vi "信号光谱9 - MoO3.vi"() -> ()   [LabVIEW 2018]
uses:
  <vilib>/Utility/NIReport.llb/Report Type.ctl
  <vilib>/Utility/file.llb/Write Delimited Spreadsheet (DBL).vi
  <vilib>/Instr/_visa.llb/VISA Configure Serial Port (Instr).vi
  <vilib>/addons/_office/excel.llb/Excel Get Data ([str]).vi
  <vilib>/Utility/NIReport.llb/NI_report.lvclass
  <vilib>/Analysis/NI_AALBase.lvlib
  <vilib>/ptbypt/NI_PtbyPt.lvlib
  <vilib>/Utility/NIReport.llb/NI_ReportGenerationCore.lvlib
  <vilib>/addons/_office/NI_ReportGenerationToolkit.lvlib
  <vilib>/Utility/NIReport.llb/Excel/NI_Excel.lvclass
panel:
  in  "判断角度上限":dbl=4.0 format="%#_13g"
  in  "判断角度下限":dbl=1.0 format="%#_13g"
  out "原始峰值":dbl
  out "拟合峰值":dbl
  in  "角度倍乘系数":dbl=1.5
  out "结果展示":dbl[][](array[numeric])=[[37.33100777239877, 2672.955043835526, 29.54153292599307, 222755.0, 50.0], [37.36593979472361, 2672.656498058864, 30.113284142729572, 222833.0, 50.0], [38.96986225690859, 2673.3337152325566, 33.38805102415213, 222910.0, 75.0], [37.39946104045098, 2676.4005085744548, 31.215565446104666, 222948.0, 47.0], [35.862209164247574, 2671.7826876859012, 30.355582265151796, 223028.0, 47.0]]
  out "Δw2>C":bool=TRUE
  out "Δw1>C":bool=TRUE
  out "θi":dbl
  in  "w0":dbl format="%#_13g"
  in  "C=w-w0":dbl=1800.0 format="%#_13g"
  in  "上升下降沿/s":dbl format="%.2p"
  in  "延时/s":dbl format="%.2p"
  in  "占空比/%":dbl=3.0 format="%.2p"
  in  "高电平/V":dbl=4.0 format="%.2p"
  in  "频率/Hz":dbl=6000.0 format="%.3p"
  in  "低电平/V":dbl min=0.0 max=5.0 format="%.2p"
  in  "Enable":bool
  in  "上升下降沿":i32(ring)=1 items=["上升沿", "下降沿"]
  in  "输出信号波形":u16(ring) items=["Pulse"]
  out "Output":bool
  in  "VISA 信号发生器":refnum<visa-resource-name>="USB0::0x1AB1::0x0641::DG4E192200870::INSTR"
  out "Output 2":bool
  in  "Enable 2":bool
  in  "上升下降沿/s 2":dbl format="%.2p"
  in  "延时/s 2":dbl format="%.2p"
  in  "占空比/% 2":dbl=3.0 format="%.2p"
  in  "高电平/V 2":dbl=0.002 format="%.2p"
  in  "频率/Hz 2":dbl=6000.0 format="%.3p"
  in  "低电平/V 2":dbl min=0.0 max=5.0 format="%.2p"
  in  "上升下降沿 2":i32(ring)=1 items=["上升沿", "下降沿"]
  in  "输出信号波形 2":u16(ring) items=["Pulse"]
  in  "终止测量":bool
  in  "测量次数":i32=1
  out "best fit":cluster{"Y":dbl[], "Y":dbl[]}[](graph)
  in  "拟合终点":i32=850
  in  "拟合起点":i32=200
  out "angle":dbl
  out "图片地址":string
  in  "开光时间/ms":u32=50
  out "最终存储路径 2":path
  out "照明光error out":errorcluster
  in  "照明光":bool
  in  "stop bits (10: 1 bit)":u16(ring)=10 items=["1.0"=10, "1.5"=15, "2.0"=20]
  in  "parity (0:none)":enum16{"None", "Odd", "Even", "Mark", "Space"}(ring)
  in  "data bits (8)":u16=8 min=5 max=8 step=1
  in  "baud rate":u32=9600 caption="baud rate (115200)" min=9600 max=115200
  in  "照明光VISA":refnum<visa-resource-name>="COM6"
  out "正在测量":bool
  in  "滤波阈值":dbl=300.0 format="%#_13g"
  out "范围内？":bool[](array[boolean])
  out "w":dbl
  out "xc":dbl
  out "拟合参数":dbl[](array[numeric])
  out "最终存储路径":path
  in  "停止程序":bool
  out "configure error out":errorcluster
  in  "设置参数":bool
  out "output control error  4":errorcluster
  in  "低电平持续输出":bool
  out "output control error  5":errorcluster
  out "output control error":errorcluster
  in  "开始测量":bool
  in  "channel输出口":i32(ring) items=["Channel 1", "Channel 2"]
  out "output control error":errorcluster
  out "Spectrum":cluster{"Y":dbl[], "Y":dbl[]}[](graph)
  out "波长范围":dbl[](array[numeric])
  in  "?":enum32{"IHR 550", "CCD"}(tab)
  in  "Move To\nTarget Positions":bool
  out "Current UniqueID":string="Mono4"
  in  "Mono ID":string(combo)="Mono1"
  in  "Connect":bool
  out "Initialized JY":bool=TRUE
  in  "Force\nInitialization":bool
  in  "Target Grating":string(combo)="2"
  out "Current Description":string="1" caption="Description"
  out "Grating Index":i32=1
  out "Current Grating":dbl=1200.0
  out "Units":string="nm"
  out "Current WL":dbl=897.9988
  out "Exit Mirror\nPosition":i32(ring)=2 items=["EntranceMirror", "ExitMirror", "Front", "Side"]
  out "Entrance Mirror\nPosition":i32(ring)=2 items=["EntranceMirror", "ExitMirror", "Front", "Side"]
  out "Units 2":string="mm"
  out "Front Entrance":dbl
  in  "Target WL":dbl=516.0
  in  "Exit Mirror":u16(ring)=3 caption="Target Position Exit Mirror" items=["Front"=2, "Side"=3]
  in  "Entrance Mirror":u16(ring)=2 caption="Target Position\nEntrance Mirror" items=["Front"=2, "Side"=3]
  in  "Target\nFront Entrance":dbl=2.0
  in  "Commande tab":T1(tab)
  in  "Area Number to Display":i32
  in  "Reformat":bool
  in  "GAIN":u16(ring)=2 caption="Device Name" items=["High Light", "Best Dynamic Range", "High Sensitivity"]
  in  "ADC":u16(ring) caption="Device Name" items=["20 kHz       ", " 1 MHz       ", " 1 MHz Ultra "]
  in  "Number of Areas :":u16=1 min=1 step=1
  in  "Integration time (ms) :":i16=20000
  out "Uniques ID":u16(ring) items=["CCD1", "CCD2"]
  in  "Device Name":u16(ring) items=["Synapse CCD (Lateral)", "Synapse_IGA (Axial)"]
  in  "Signal type :":enum16{"TTL Rising Edge", "TTL Falling Edge"}(ring)=enum."TTL Falling Edge"
  in  "Trigger Type :":u16(ring) items=["On Start"=1, "Per Acquisition"=2]
  in  "trigSigTypeString":string
  in  "trigEventString":string
  in  "Enable InputTriggers :":bool
  in  "Number of Cleans":i32=1
  in  "MultiAcqShutterMode":i32(ring)=3 items=["Open For All Spectra"=1, "Open for Each Spectrum"=3]
  in  "Accumulations:":u16=10 min=1 step=1
  in  "Multi Accumulation mode:":bool
  out "Y Pixels:":i32=256
  out "DataSize":i32=1024
  out "X Pixels:":i32=1024
  out "Firmware\nVersion":string="V1.20 CCD_4000"
  out "initialized ?":bool=TRUE
  in  "Continuous":bool
  in  "CCD Busy":bool
  out "indicator":string="Ready !"
  in  "initialize":bool
  in  "ShutterOpen":bool=TRUE caption="Shutter enable"
  in  "Acquire":bool
  in  "Temperature":bool
  in  "Setup":bool
  out "Acq Time(ms)":u32=3401
  in  "Save Backlight":bool
  in  "cut backlight":bool
  out "backlight":bool=TRUE
  in  "是否拟合":bool
  in  "是否保存":bool
  in  "Close":bool=TRUE
  out "JYCCDLib.IJYCCDReqd":refnum<k7>
  out "areas :":i32[][](array[numeric])=[[1], [1], [1], [1024], [256], [1], [256]]
  in  "Constante de condition\n(Voir l'aide contextuelle)":bool
  out "temp graph":dbl(graph)=-134.538067
  out "ADC Number":i32[](array[numeric])=[0, 1, 2, 3, 4]
  out "Gain Number":i32[](array[numeric])=[10, 11, 12, 13, 8, 2]
  out "trigAddress":i32
  out "Data":i32[][](graph)
  out "error out":errorcluster
  out "Gratings":dbl[](array[numeric])=[1200.0, 300.0]
  out "Backlight":i32[][](graph)
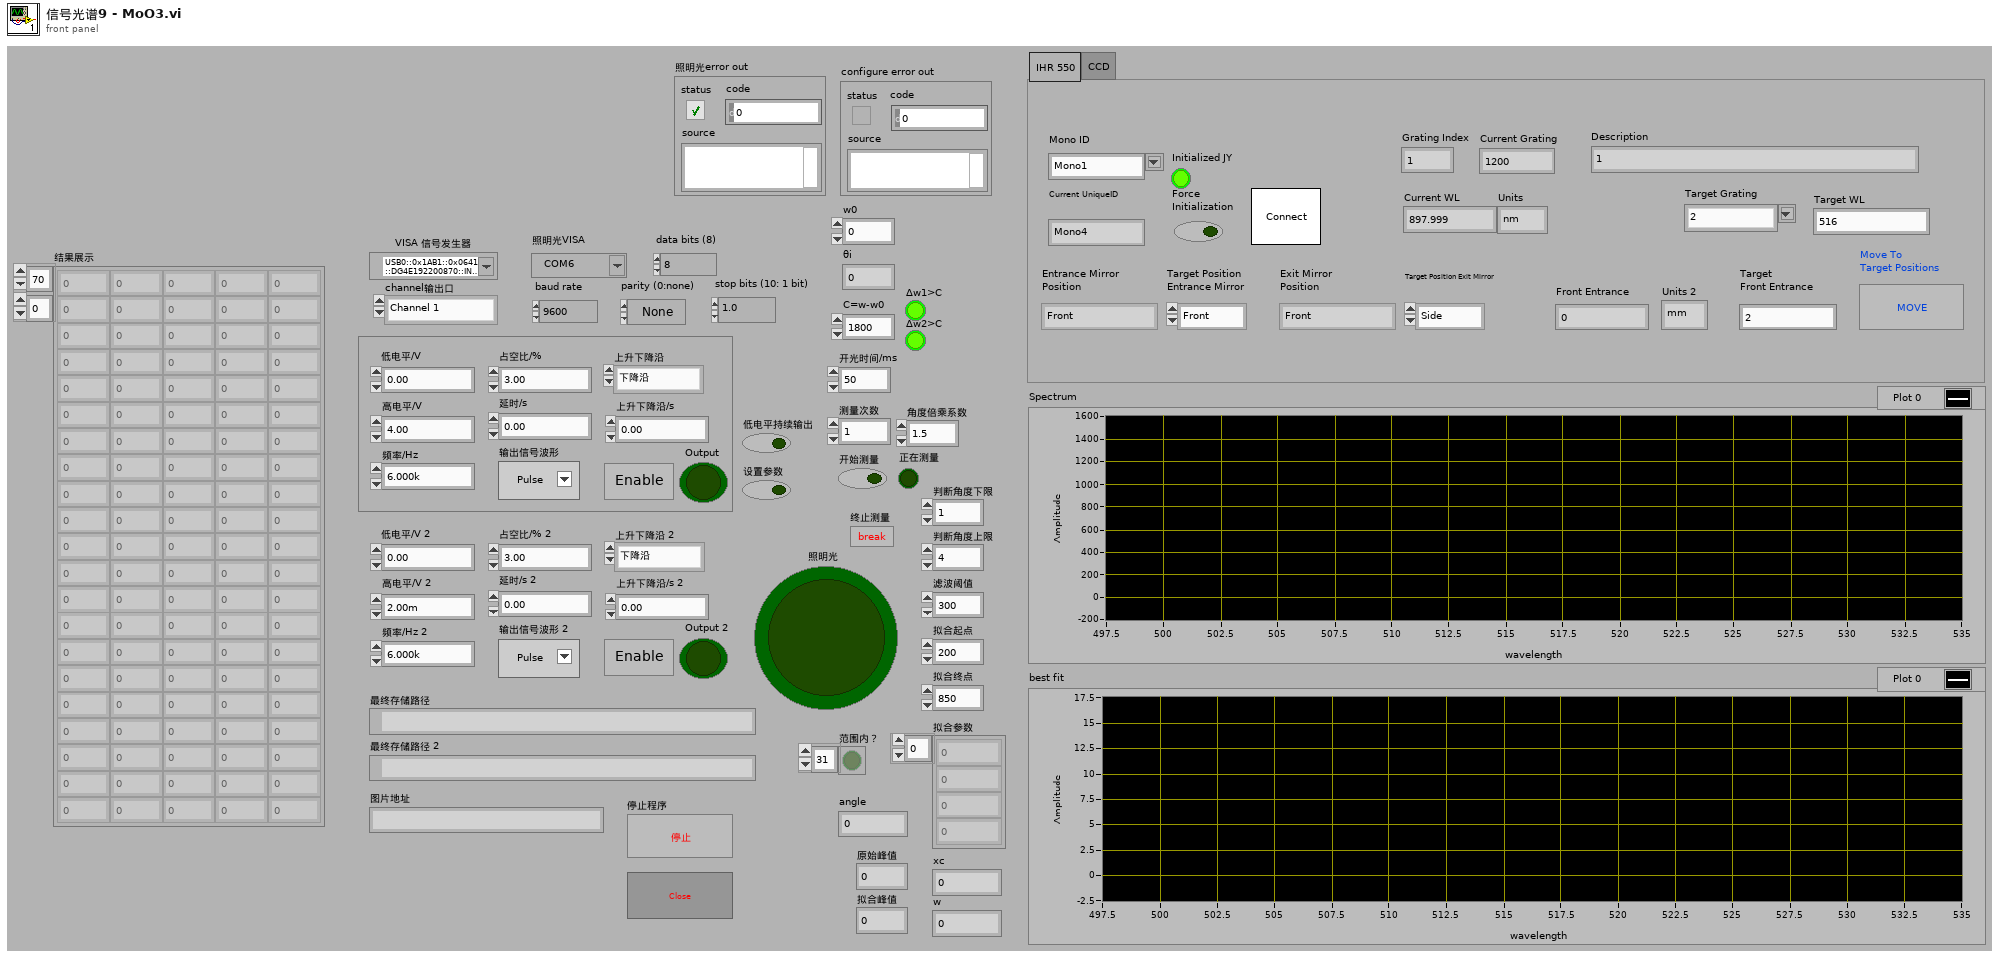
[diagram p1: front panel]
types:
  T1 = enum32{"Settings", "Trigger In", "Multi-Accu.", "Infos"}
  T2 = enum8{"Enabled", "Disabled", "Disabled and Grayed Out"}
  T3 = enum16{"maximized", "minimized", "normal", "no change"}
  T4 = typedef "NI_ReportGenerationCore.lvlib/Report Type.ctl" = enum16{"HTML", "Word", "Excel"}
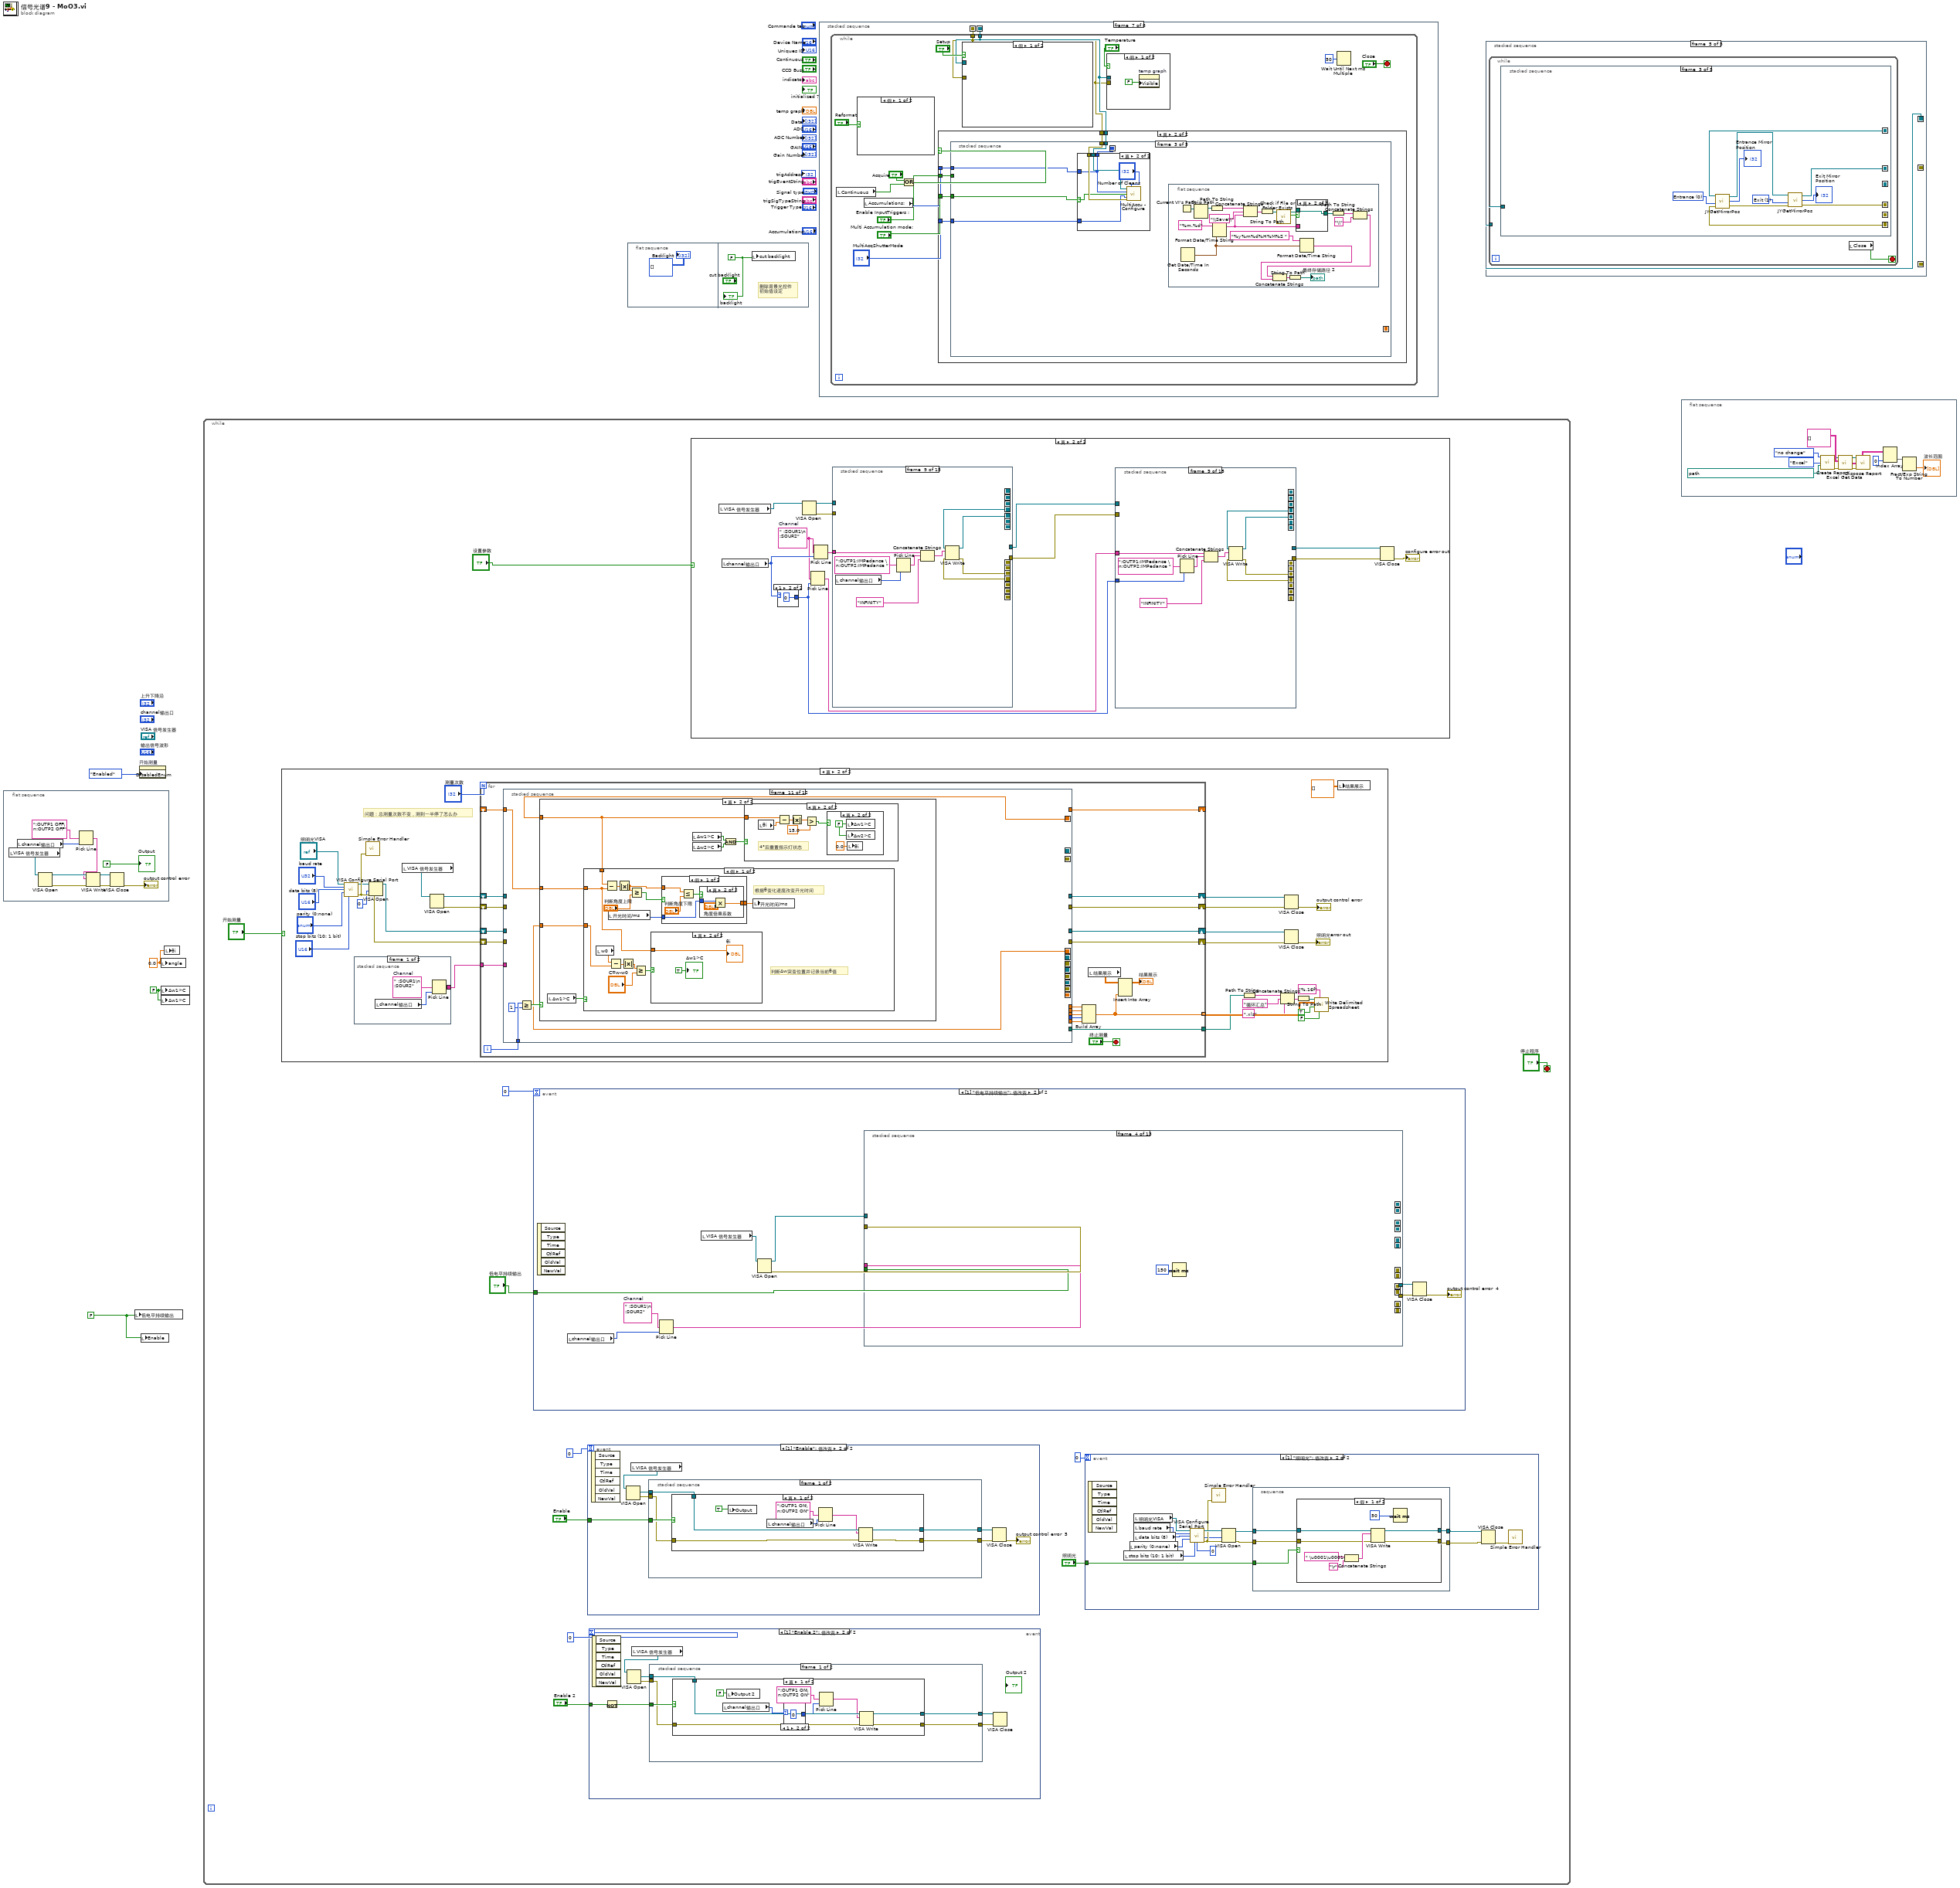
[diagram p0: block diagram]
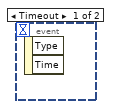
[diagram p2: hidden frame]
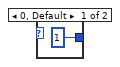
[diagram p3: hidden frame]
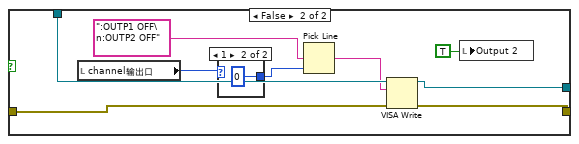
[diagram p4: hidden frame]
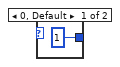
[diagram p5: hidden frame]
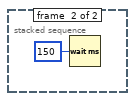
[diagram p6: hidden frame]
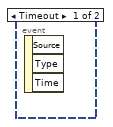
[diagram p7: hidden frame]
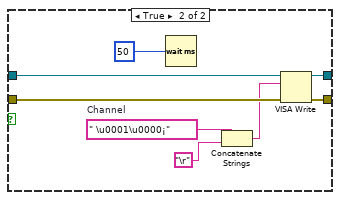
[diagram p8: hidden frame]
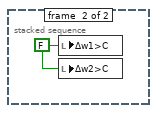
[diagram p10: hidden frame]
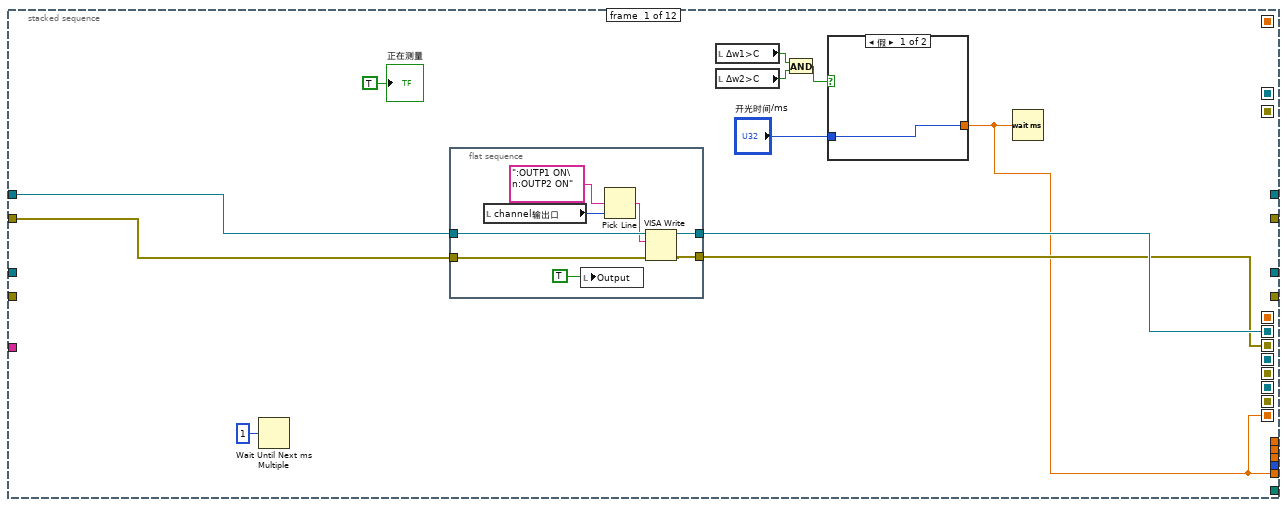
[diagram p11: hidden frame]
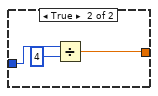
[diagram p12: hidden frame]
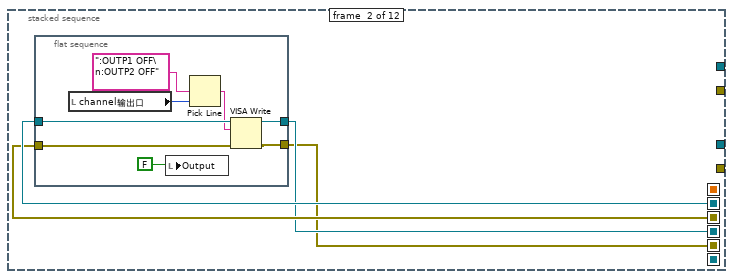
[diagram p13: hidden frame]
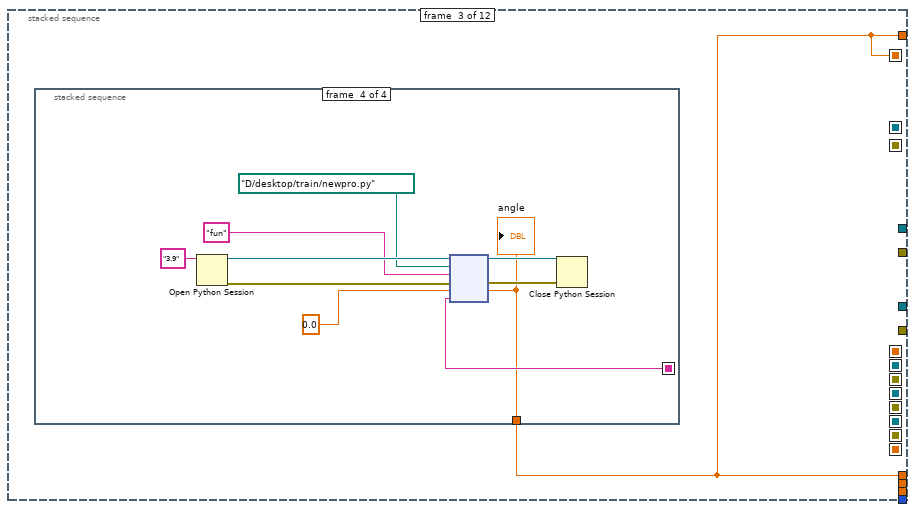
[diagram p14: hidden frame]
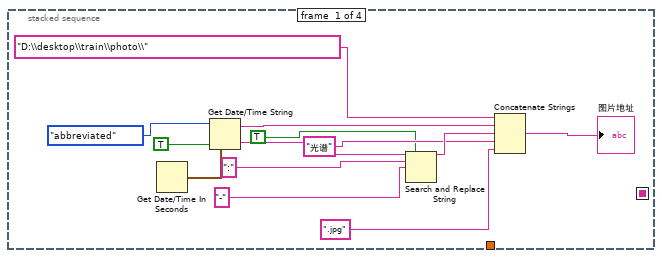
[diagram p15: hidden frame]
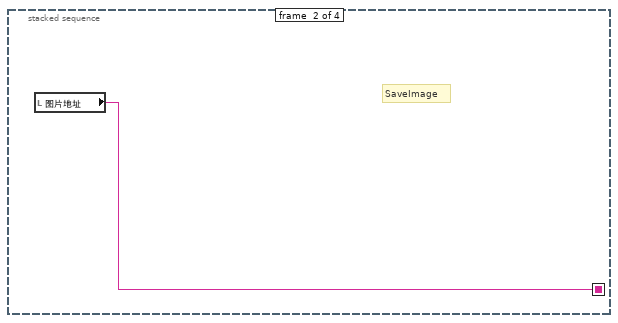
[diagram p16: hidden frame]
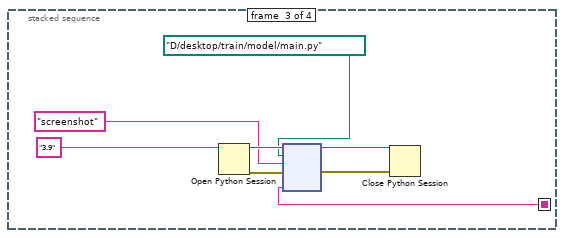
[diagram p17: hidden frame]
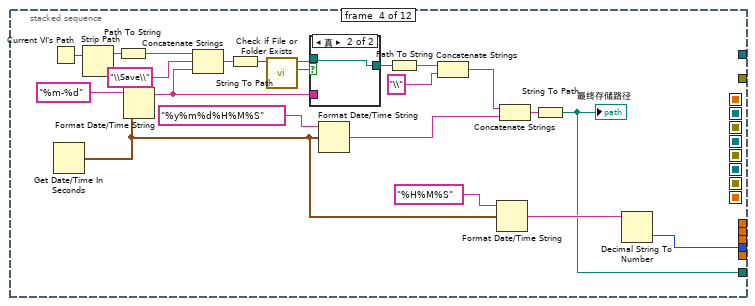
[diagram p18: hidden frame]
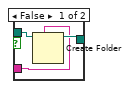
[diagram p19: hidden frame]
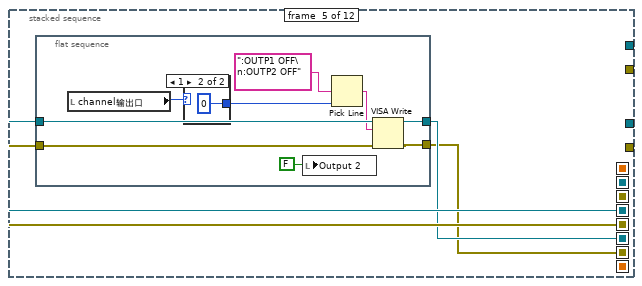
[diagram p20: hidden frame]
diagram:
  w1 = FALSE ("Δw1>C")
  w2 = 0.0 ("angle")
  w3 = FALSE
  n1 = flat-sequence {
    frame #0 {
      n2 = local read "VISA 信号发生器"() -> (w8:refnum<visa-resource-name>)
      n3 = local read "channel输出口"() -> (w6:i32)
      n4 = VISA Open(VISA resource name=w8) -> (VISA resource name=w14:refnum<visa-resource-name>, error out=w13:errorcluster)  [unwired: 4 in]
      n5 = Pick Line(multi-line string=":OUTP1 OFF\n:OUTP2 OFF" ("write buffer"), line index=w6) -> (output string=w5:string)  [unwired: 1 in]
      n6 = VISA Write(VISA resource name=w14, write buffer=w5, error in (no error)=w13) -> (VISA resource name out=w11:refnum<visa-resource-name>, error out=w10:errorcluster)  [unwired: 1 out]
      n7 = VISA Close(VISA resource name=w11, error in (no error)=w10) -> (error out=→"output control error":errorcluster)
      "Output" <- FALSE ("布尔")
    }
  }
  n8 = local write "低电平持续输出"(w3) -> ()
  n9 = property on="开始测量" class="Bool"("DisabledEnum"=T2."Enabled" ("禁用")) -> ()  [unwired: 2 in, 2 out]
  n10 = local write "Enable"(w3) -> ()
  n11 = local write "angle"(w2) -> ()
  n12 = local write "Δw1>C"(w1) -> ()
  n13 = local write "Δw1>C"(w1) -> ()
  n14 = local write "θi"(w2) -> ()
  n15 = while {
    stop <- "停止程序" stop-if-true
    n16 = case shown="真" "开始测量" {
      frame False {
      }
      frame True {
        # "问题：总测量次数不变，测到一半停了怎么办"
        n17 = call-poly "VISA Configure Serial Port"("VISA resource name"="照明光VISA", "baud rate (9600)"="baud rate", "data bits (8)"="data bits (8)", "parity (0:none)"="parity (0:none)", "stop bits (10: 1 bit)"="stop bits (10: 1 bit)") -> ("VISA resource name out"=w118:refnum<visa-resource-name>, "error out"=w119:errorcluster)  [unwired: 9 in]
        n18 = stacked-sequence {
          tunnel: [w128 _] -> w122
          frame #0 {
            w129 = " :SOUR1\n :SOUR2"  # Channel
            n19 = local read "channel输出口"() -> (w130:i32)
            n20 = Pick Line(multi-line string=w129, line index=w130) -> (output string=w128:string)  [unwired: 1 in]
          }
          frame #1 {
            w131 = FALSE ("Δw1>C")
            n21 = local write "Δw1>C"(w131) -> ()
            n22 = local write "Δw2>C"(w131) -> ()
          }
        }
        n23 = call <vilib>:"Simple Error Handler.vi"("error in (no error)"=w119) -> ()  [unwired: 4 in, 5 out]
        n24 = VISA Open(access mode=0, error in (no error)=w119, VISA resource name=w118) -> (VISA resource name=w111:refnum<visa-resource-name>, error out=w110:errorcluster)  [unwired: 2 in]
        n25 = local read "VISA 信号发生器"() -> (w127:refnum<visa-resource-name>)
        n26 = VISA Open(VISA resource name=w127) -> (VISA resource name=w126:refnum<visa-resource-name>, error out=w125:errorcluster)  [unwired: 4 in]
        n27 = for {
          N: "测量次数" -> [_]
          tunnel: w122 -> [w151]
          shift-right: [w147] -> w121
          shift-left: w126 -> [w153]
          shift-right: [w146] -> w120
          shift-left: w125 -> [w152]
          shift-right: [w145] -> w124
          shift-left: w111 -> [w150]
          shift-right: [w144] -> w123
          shift-left: w110 -> [w149]
          tunnel: [w134] -> w100 mode=indexing
          shift-right: [w139] -> _
          shift-left: _ -> [w138]
          tunnel: [w135] -> w97
          i -> [w137]
          stop <- "终止测量" stop-if-true
          n28 = stacked-sequence {
            seq-local: [w160 _ _ _ _ _ _ _ _ _ _ _] -> [_ w180 _ _ _ _ _ _ _ _ _ _]
            seq-local: [w159 _ _ _ _ _ _ _ _ _ _ _] -> [_ w179 _ _ _ _ _ _ _ _ _ _]
            seq-local: [_ _ _ _ _ w265 _ _ _ _ _ _] -> [_ _ _ _ _ _ _ _ w383 _ _ _]
            seq-local: [_ _ _ _ _ w264 _ _ _ _ _ _] -> [_ _ _ _ _ _ _ _ w386 _ _ _]
            seq-local: [_ w178 _ _ _ _ _ _ _ _ _ _] -> [_ _ _ _ w251 _ _ _ _ _ _ _]
            seq-local: [_ w177 _ _ _ _ _ _ _ _ _ _] -> [_ _ _ _ w250 _ _ _ _ _ _ _]
            seq-local: [_ _ _ _ w249 _ _ _ _ _ _ _] -> [_ _ _ _ _ _ _ w369 _ _ _ _]
            seq-local: [_ _ _ _ w248 _ _ _ _ _ _ _] -> [_ _ _ _ _ _ _ w368 _ _ _ _]
            seq-local: [_ _ w189 _ _ _ _ _ _ _ _ _] -> [_ _ _ _ _ _ _ _ _ _ w395 _]
            seq-local: [_ _ _ _ _ _ w280 _ _ _ _ _] -> [_ _ _ _ _ _ _ _ _ _ w390 _]
            seq-local: [w154 _ _ _ _ _ _ _ _ _ _ _] -> [_ _ _ _ _ _ w278 _ _ _ _ _]
            tunnel: w153 -> [w162 _ _ _ _ _ _ _ _ _ _ _]
            tunnel: w152 -> [w161 _ _ _ _ _ _ _ _ _ _ _]
            tunnel: [_ _ _ _ _ _ _ w367 _ _ _ _] -> w147
            tunnel: [_ _ _ _ _ _ _ w366 _ _ _ _] -> w146
            tunnel: w151 -> [_ _ _ _ _ _ _ _ _ _ _ _]
            tunnel: w150 -> [_ _ _ _ _ w268 _ _ _ _ _ _]
            tunnel: w149 -> [_ _ _ _ _ w267 _ _ _ _ _ _]
            tunnel: [_ _ _ _ _ _ _ _ w385 _ _ _] -> w145
            tunnel: [_ _ _ _ _ _ _ _ w384 _ _ _] -> w144
            tunnel: [_ _ w189 _ _ _ _ _ _ _ _ _] -> w143
            tunnel: [_ _ _ _ _ _ w275 _ _ _ _ _] -> w142
            tunnel: [_ _ _ _ _ _ w274 _ _ _ _ _] -> w141
            tunnel: [_ _ _ w223 _ _ _ _ _ _ _ _] -> w140
            tunnel: [w154 _ _ _ _ _ _ _ _ _ _ _] -> w136
            tunnel: [_ _ w189 _ _ _ _ _ _ _ _ _] -> w139
            tunnel: w138 -> [_ _ _ _ _ _ _ _ _ _ w394 _]
            tunnel: w137 -> [_ _ _ _ _ _ _ _ _ _ w392 _]
            tunnel: [_ _ _ w222 _ _ _ _ _ _ _ _] -> w135
            frame #0 {
              n29 = Wait Until Next ms Multiple(millisecond multiple=u32 1 ("毫秒倍数")) -> ()  [unwired: 1 out]
              n30 = flat-sequence {
                tunnel: w162 -> [w176]
                tunnel: w161 -> [w175]
                tunnel: [w170] -> w160
                tunnel: [w169] -> w159
                frame #0 {
                  n31 = local read "channel输出口"() -> (w172:i32)
                  n32 = local write "Output"(TRUE ("布尔")) -> ()
                  n33 = Pick Line(multi-line string=":OUTP1 ON\n:OUTP2 ON" ("write buffer"), line index=w172) -> (output string=w171:string)  [unwired: 1 in]
                  n34 = VISA Write(VISA resource name=w176, write buffer=w171, error in (no error)=w175) -> (VISA resource name out=w170:refnum<visa-resource-name>, error out=w169:errorcluster)  [unwired: 1 out]
                }
              }
              n35 = local read "Δw1>C"() -> (w156:bool)
              n36 = local read "Δw2>C"() -> (w157:bool)
              n37 = And(x=w156, y=w157) -> (x .and. y?=w155:bool)
              n38 = case shown="假" w155 {
                tunnel: [w165 w166] -> w154
                tunnel: "开光时间/ms" -> [w165 w168]
                frame False {
                }
                frame True {
                  n39 = Divide(x=w168, y=u32 4) -> (x/y=w166:dbl)
                }
              }
              n40 = Wait (ms)(milliseconds to wait=w154) -> ()  [unwired: 1 out]
              "正在测量" <- TRUE
            }
            frame #1 {
              n41 = flat-sequence {
                tunnel: w180 -> [w188]
                tunnel: w179 -> [w187]
                tunnel: [w182] -> w178
                tunnel: [w181] -> w177
                frame #0 {
                  n42 = local read "channel输出口"() -> (w184:i32)
                  n43 = local write "Output"(FALSE ("布尔")) -> ()
                  n44 = Pick Line(multi-line string=":OUTP1 OFF\n:OUTP2 OFF" ("write buffer"), line index=w184) -> (output string=w183:string)  [unwired: 1 in]
                  n45 = VISA Write(VISA resource name=w188, write buffer=w183, error in (no error)=w187) -> (VISA resource name out=w182:refnum<visa-resource-name>, error out=w181:errorcluster)  [unwired: 1 out]
                }
              }
            }
            frame #2 {
              n46 = stacked-sequence {
                seq-local: [_ w203 _ _] -> [_ _ w204 w213]
                tunnel: [_ _ _ w212] -> w189
                frame #0 {
                  n47 = Get Date/Time In Seconds() -> (seconds since 1Jan1904=w199:timestamp)
                  n48 = Get Date/Time String(date format (0)=enum16{"short", "long", "abbreviated"}."abbreviated" ("日期格式(0)"), seconds (now)=w199, want seconds? (F)=TRUE ("需要秒？(F)")) -> (date string=w202:string, time string=w200:string)
                  n49 = Search and Replace String(replace all?=TRUE ("替换全部？(F)"), input string=w200, search string=":" ("搜索字符串"), replace string="-" ("替换字符串(\"\")")) -> (result string=w201:string)  [unwired: 4 in, 3 out]
                  n50 = Concatenate Strings("D:\\desktop\\train\\photo\\", w202, w201, "光谱" ("字符串"), ".jpg" ("字符串")) -> (→"图片地址":string)
                }
                frame #1 {
                  # "SaveImage"
                  n51 = local read "图片地址"() -> (w203:string)
                }
                frame #2 {
                  n52 = Open Python Session(python version="3.9" ("Python version")) -> (session out=w211:refnum<k35>, error out=w209:errorcluster)  [unwired: 2 in]
                  n53 = node(w211, path "D:/desktop/train/model/main.py" ("module path"), "screenshot" ("function name"), w209, w204) -> (w210:refnum<k35>, w208:errorcluster)  [unwired: 3 in, 2 out]
                  n54 = Close Python Session(session in=w210, error in=w208) -> ()  [unwired: 1 out]
                }
                frame #3 {
                  n55 = Open Python Session(python version="3.9" ("Python version")) -> (session out=w220:refnum<k35>, error out=w218:errorcluster)  [unwired: 2 in]
                  n56 = node(w220, path "D:/desktop/train/newpro.py" ("module path"), "fun" ("function name"), w218, 0.0, w213) -> (w219:refnum<k35>, w217:errorcluster, w212:dbl)  [unwired: 1 in, 2 out]
                  "angle" <- w212
                  n57 = Close Python Session(session in=w219, error in=w217) -> ()  [unwired: 1 out]
                }
              }
            }
            frame #3 {
              n58 = Current VI's Path() -> (path=w232:path)
              n59 = Get Date/Time In Seconds() -> (seconds since 1Jan1904=w225:timestamp)
              n60 = Strip Path(path=w232) -> (stripped path=w233:path)  [unwired: 1 out]
              n61 = Path To String(path=w233) -> (string=w234:string)
              n62 = Format Date/Time String(time format string (%c)="%m-%d" ("时间格式字符串(%c)"), seconds (now)=w225) -> (date/time string=w240:string)  [unwired: 1 in]
              n63 = Concatenate Strings(w234, "\\Save\\" ("字符串"), w240) -> (w235:string)
              n64 = String To Path(string=w235) -> (path=w236:path)
              n65 = call <vilib>:"Check if File or Folder Exists.vi"("path"=w236) -> ("file or folder exists?"=w237:bool, "dup path"=w239:path)  [unwired: 8 in, 1 out]
              n66 = case shown="真" w237 {
                tunnel: [w246 w247] -> w238
                tunnel: w239 -> [w245 w247]
                tunnel: w240 -> [w244 _]
                frame False {
                  n67 = Create Folder(prompt (Create Folder)=w244, path (use dialog)=w245) -> (created path=w246:path)  [unwired: 1 in, 2 out]
                }
                frame True {
                }
              }
              n68 = Format Date/Time String(time format string (%c)="%y%m%d%H%M%S" ("时间格式字符串(%c)"), seconds (now)=w225) -> (date/time string=w243:string)  [unwired: 1 in]
              n69 = Path To String(path=w238) -> (string=w241:string)
              n70 = Concatenate Strings(w241, "\\" ("字符串")) -> (w242:string)
              n71 = Format Date/Time String(time format string (%c)="%H%M%S" ("时间格式字符串(%c)"), seconds (now)=w225) -> (date/time string=w224:string)  [unwired: 1 in]
              n72 = Concatenate Strings(w242, w243) -> (w231:string)
              n73 = String To Path(string=w231) -> (path=w222:path)
              "最终存储路径" <- w222
              n74 = Decimal String To Number(string=w224) -> (number=w223:i32)  [unwired: 2 in, 1 out]
            }
            frame #4 {
              n75 = flat-sequence {
                tunnel: w251 -> [w260]
                tunnel: w250 -> [w259]
                tunnel: [w255] -> w249
                tunnel: [w254] -> w248
                frame #0 {
                  n76 = local read "channel输出口"() -> (w253:i32)
                  n77 = case shown="1" w253 {
                    tunnel: [1 0] -> w252
                    frame 0, Default {
                    }
                    frame 1 {
                    }
                  }
                  n78 = local write "Output 2"(FALSE ("布尔")) -> ()
                  n79 = Pick Line(multi-line string=":OUTP1 OFF\n:OUTP2 OFF" ("write buffer"), line index=w252) -> (output string=w256:string)  [unwired: 1 in]
                  n80 = VISA Write(VISA resource name=w260, write buffer=w256, error in (no error)=w259) -> (VISA resource name out=w255:refnum<visa-resource-name>, error out=w254:errorcluster)  [unwired: 1 out]
                }
              }
            }
            frame #5 {
              w263 = " \u0001\u0001¢"  # Channel
              n81 = Wait (ms)(milliseconds to wait=1200) -> ()  [unwired: 1 out]
              n82 = Concatenate Strings(w263, "\r") -> (w269:string)
              n83 = local write "照明光"(FALSE ("照明光")) -> ()
              n84 = VISA Write(VISA resource name=w268, write buffer=w269, error in (no error)=w267) -> (VISA resource name out=w265:refnum<visa-resource-name>, error out=w264:errorcluster)  [unwired: 1 out]
            }
            frame #6 {
              n85 = local read "Area Number to Display"() -> (w319:i32)
              n86 = local read "JYCCDLib.IJYCCDReqd"() -> (w315:refnum<k7>)
              n87 = Get Date/Time In Seconds() -> (seconds since 1Jan1904=w328:timestamp)
              n88 = local read "最终存储路径"() -> (w342:path)
              n89 = Get Date/Time String(date format (0)=enum16{"short", "long", "abbreviated"}."abbreviated" ("日期格式(0)"), seconds (now)=w328, want seconds? (F)=TRUE ("需要秒？(F)")) -> (date string=w336:string, time string=w331:string)
              n90 = call "MultiAccu - Acquire spectral.vi"("error in"=errorcluster {"status"=FALSE, "code"=0, "source"=""}, "Accumulations:"=u16 1, "ShutterOpen"=TRUE, "JYCCDLib.IJYCCDReqd"=w315) -> ("Acq Time(ms)"=w321:u32, "Array Out"=w320:i32[][][])  [unwired: 1 out]
              n91 = local write "Acq Time(ms)"(w321) -> ()
              n92 = local read "cut backlight"() -> (w303:bool)
              n93 = local read "backlight"() -> (w301:bool)
              n94 = Search and Replace String(replace all?=TRUE ("替换全部？(F)"), input string=w331, search string=":" ("搜索字符串"), replace string="-" ("替换字符串(\"\")")) -> (result string=w335:string)  [unwired: 4 in, 3 out]
              n95 = Path To String(path=w342) -> (string=w325:string)
              n96 = And(x=w303, y=w301) -> (x .and. y?=w302:bool)
              n97 = call "Array reset dimension.vi"("Area Number"=w319, "Array In"=w320) -> ("Array Out"=w305:i32[][])
              n98 = Concatenate Strings(w325, w336, w335, "光谱" ("字符串"), ".xls" ("字符串")) -> (w340:string)
              n99 = case shown="真" w302 {
                tunnel: [w362 w364] -> w304
                tunnel: w305 -> [w362 w363]
                frame False {
                }
                frame True {
                  n100 = local read "Backlight"() -> (w365:i32[][])
                  n101 = Subtract(x=w363, y=w365) -> (x-y=w364:i32[][])
                }
              }
              n102 = String To Path(string=w340) -> (path=w341:path)
              n103 = local write "Data"(w305) -> ()
              n104 = local read "波长范围"() -> (w273:dbl[])
              n105 = Index Array(array=w304, index (row)=0 ("索引 (行)")) -> (element=w343:i32[])  [unwired: 1 in]
              n106 = Reverse 1D Array(array=w343) -> (reversed array=w272:i32[])
              n107 = local read "angle"() -> (w284:dbl)
              n108 = local read "拟合起点"() -> (w291:i32)
              n109 = local read "拟合终点"() -> (w293:i32)
              n110 = call <vilib>:"Median Filter.vi"("left rank"=6, "X"=w272) -> ("Filtered X"=w282:dbl[])  [unwired: 8 in, 1 out]
              n111 = Build Array(w284, w278, 0.0 ("元素")) -> (w283:dbl[])
              n112 = Subtract(x=w293, y=w291) -> (x-y=w290:i32)
              n113 = call "Convert to Dynamic Data"("Array"=w273) -> ("Dynamic Data Type"=w312:dynamicdata)  [unwired: 3 in]
              n114 = call "Convert to Dynamic Data2"("Array"=w272) -> ("Dynamic Data Type"=w311:dynamicdata)  [unwired: 3 in]
              n115 = Array Subset(array=w273, index=w291, length=w290) -> (w289:dbl[])
              n116 = call "Build XY Graph"("Y Input"=w311, "X Input"=w312) -> ("XY Graph"=→"Spectrum":cluster{"Y":dbl[], "Y":dbl[]}[])  [unwired: 8 in, 1 out]
              n117 = call "转换至动态数据4"("Array"=w289) -> ("Dynamic Data Type"=w309:dynamicdata)  [unwired: 3 in]
              n118 = In Range and Coerce(upper limit="滤波阈值", x=w282, lower limit=-100.0) -> (In Range?=w296:bool[])  [unwired: 1 out]
              "范围内？" <- w296
              n119 = Not(x=w296) -> (.not. x?=w295:bool[])
              n120 = Or Array Elements(Boolean array=w295) -> (logical OR=w298:bool)
              n121 = local read "X Pixels:"() -> (w297:i32)
              n122 = local read "波长范围"() -> (w285:dbl[])
              n123 = local read "滤波阈值"() -> (w294:dbl)
              n124 = case shown="真" w298 {
                tunnel: w297 -> [_ w349]
                tunnel: w282 -> [w345 w348]
                tunnel: [w345 w347] -> w276
                tunnel: w294 -> [_ w346]
                frame False {
                }
                frame True {
                  n125 = for {
                    N: w349 -> [_]
                    tunnel: w348 -> [w353] mode=indexing
                    tunnel: [w352] -> w347 mode=indexing
                    shift-right: [w352] -> _
                    shift-left: _ -> [w351]
                    tunnel: w346 -> [w350]
                    n126 = Greater?(x=w353, y=w350) -> (0:w355:bool)
                    n127 = Less?(x=w353, y=-100.0) -> (x < y?=w356:bool)
                    n128 = Or(x=w355, y=w356) -> (x .or. y?=w354:bool)
                    n129 = case shown="真" w354 {
                      tunnel: w353 -> [w358 _]
                      tunnel: [w358 w360] -> w352
                      tunnel: w351 -> [_ w361]
                      frame False {
                      }
                      frame True {
                        n130 = call <vilib>:"Median Filter PtByPt.vi"("rank"=5, "x"=w361) -> ("Filtered x"=w360:dbl)  [unwired: 2 in, 1 out]
                      }
                    }
                  }
                }
              }
              n131 = Array Subset(array=w276, index=w291, length=w290) -> (w292:dbl[])
              n132 = call "转换至动态数据3"("Array"=w292) -> ("Dynamic Data Type"=w310:dynamicdata)  [unwired: 3 in]
              n133 = call "曲线拟合"("Locations"=w309, "Signals"=w310) -> ("best fit"=w314:dynamicdata, "non-linear coefficients"=w313:dynamicdata)  [unwired: 5 in, 3 out]
              n134 = call "从动态数据转换"("Dynamic Data Type"=w313) -> ("Array"=w306:dbl[])  [unwired: 3 in]
              "拟合参数" <- w306
              n135 = call "从动态数据转换2"("Dynamic Data Type"=w314) -> ("Array"=w277:dbl[])  [unwired: 3 in]
              n136 = Build Array(w273, w272, w282, w277, w306, w283) -> (w344:dbl[][])
              n137 = call-poly <vilib>:"Write Delimited Spreadsheet.vi"("file path (dialog if empty)"=w341, "format (%.3f)"="%.16f", "2D data"=w344, "append to file? (new file:F)"=TRUE ("append to file? (F)"), "transpose? (no:F)"=TRUE ("transpose? (F)")) -> ()  [unwired: 9 in, 2 out]
              n138 = Index Array(array=w306, index #1=0 ("索引"), index #2=1 ("索引")) -> (element #1=→"xc":dbl, element #2=w280:dbl)
              "w" <- w280
              n139 = Bundle("波长范围"=w285, "Filtered X"=w276) -> (w288:cluster{"波长范围 ":dbl[], "Filtered X":dbl[]})  [unwired: 1 in]
              n140 = Bundle(w289, "Array"=w277) -> (w287:cluster{dbl[], "Array":dbl[]})  [unwired: 1 in]
              n141 = Array Max & Min(array=w277) -> (max value=w274:dbl)  [unwired: 3 out]
              "拟合峰值" <- w274
              n142 = Array Max & Min(array=w276) -> (max value=w275:dbl)  [unwired: 3 out]
              "原始峰值" <- w275
              n143 = Build Array(w288, w287) -> (w286:cluster{"波长范围 ":dbl[], "Array":dbl[]}[])
              n144 = local write "best fit"(w286) -> ()
            }
            frame #7 {
              n145 = flat-sequence {
                tunnel: w369 -> [w378]
                tunnel: w368 -> [w377]
                tunnel: [w373] -> w367
                tunnel: [w372] -> w366
                frame #0 {
                  n146 = local read "channel输出口"() -> (w371:i32)
                  n147 = case shown="1" w371 {
                    tunnel: [1 0] -> w370
                    frame 0, Default {
                    }
                    frame 1 {
                    }
                  }
                  n148 = local write "Output 2"(TRUE ("布尔")) -> ()
                  n149 = Pick Line(multi-line string=":OUTP1 ON\n:OUTP2 ON" ("write buffer"), line index=w370) -> (output string=w374:string)  [unwired: 1 in]
                  n150 = VISA Write(VISA resource name=w378, write buffer=w374, error in (no error)=w377) -> (VISA resource name out=w373:refnum<visa-resource-name>, error out=w372:errorcluster)  [unwired: 1 out]
                }
              }
            }
            frame #8 {
              w381 = " \u0001\u0000¡"  # Channel
              n151 = Concatenate Strings(w381, "\r") -> (w387:string)
              n152 = VISA Write(VISA resource name=w383, write buffer=w387, error in (no error)=w386) -> (VISA resource name out=w385:refnum<visa-resource-name>, error out=w384:errorcluster)  [unwired: 1 out]
              n153 = local write "照明光"(TRUE ("照明光")) -> ()
            }
            frame #9 {
              n154 = Wait (ms)(milliseconds to wait=900) -> ()  [unwired: 1 out]
            }
            frame #10 {
              n155 = Greater Or Equal?(x=w392, y=1) -> (x >= y?=w393:bool)
              n156 = case shown="真" w393 {
                tunnel: w395 -> [_ w401]
                tunnel: w394 -> [_ w402]
                tunnel: w390 -> [w396 w403]
                frame False {
                  n157 = local write "w0"(w396) -> ()
                }
                frame True {
                  n158 = local read "Δw1>C"() -> (w400:bool)
                  n159 = case shown="假" w400 {
                    tunnel: w403 -> [w422 w442]
                    tunnel: w402 -> [w412 _]
                    tunnel: w401 -> [w413 _]
                    frame False {
                      # "判断Δw突变位置并记录当前θ值"
                      # "根据θ变化速度改变开光时间"
                      n160 = local read "w0"() -> (w420:dbl)
                      n161 = Subtract(x=w413, y=w412) -> (x-y=w415:dbl)
                      n162 = local read "开光时间/ms"() -> (w418:u32)
                      n163 = Subtract(x=w420, y=w422) -> (x-y=w425:dbl)
                      n164 = Absolute Value(x=w415) -> (abs(x)=w417:dbl)
                      n165 = Absolute Value(x=w425) -> (abs(x)=w423:dbl)
                      n166 = Greater Or Equal?(x=w417, y="判断角度上限") -> (x >= y?=w416:bool)
                      n167 = Greater Or Equal?(x=w423, y="C=w-w0") -> (x >= y?=w421:bool)
                      n168 = case shown="真" w421 {
                        tunnel: w412 -> [_ w440]
                        frame False {
                          w438 = FALSE ("Δw1>C")
                          n169 = local write "Δw1>C"(w438) -> ()
                          n170 = local write "Δw2>C"(w438) -> ()
                        }
                        frame True {
                          "θi" <- w440
                          "Δw1>C" <- TRUE ("布尔")
                        }
                      }
                      n171 = case shown="假" w416 {
                        tunnel: w417 -> [w430 _]
                        tunnel: w418 -> [w427 w437]
                        tunnel: [w426 w435] -> w419
                        frame False {
                          n172 = Less Or Equal?(x=w430, y="判断角度下限") -> (x <= y?=w428:bool)
                          n173 = case shown="真" w428 {
                            tunnel: w427 -> [w431 w434]
                            tunnel: [w431 w433] -> w426
                            frame False {
                            }
                            frame True {
                              n174 = Multiply(x=w434, y="角度倍乘系数") -> (x*y=w433:dbl)
                            }
                          }
                        }
                        frame True {
                          n175 = Divide(x=w437, y=1.6) -> (x/y=w435:dbl)
                        }
                      }
                      n176 = local write "开光时间/ms"(w419) -> ()
                    }
                    frame True {
                      # "再次判断Δw，排除坏点影响"
                      n177 = local read "Δw2>C"() -> (w441:bool)
                      n178 = case shown="假" w441 {
                        tunnel: w442 -> [w445 _]
                        frame False {
                          n179 = local read "C=w-w0"() -> (w443:dbl)
                          n180 = local read "w0"() -> (w446:dbl)
                          n181 = Subtract(x=w446, y=w445) -> (x-y=w448:dbl)
                          n182 = Absolute Value(x=w448) -> (abs(x)=w447:dbl)
                          n183 = Greater Or Equal?(x=w447, y=w443) -> (x >= y?=w444:bool)
                          n184 = case shown="真" w444 {
                            frame False {
                              n185 = local write "θi"(0.0 ("θi")) -> ()
                              n186 = local write "Δw1>C"(FALSE ("Δw1>C")) -> ()
                            }
                            frame True {
                              "Δw2>C" <- TRUE
                            }
                          }
                        }
                        frame True {
                        }
                      }
                    }
                  }
                  n187 = local read "Δw1>C"() -> (w398:bool)
                  n188 = local read "Δw2>C"() -> (w399:bool)
                  n189 = And(x=w398, y=w399) -> (x .and. y?=w397:bool)
                  n190 = case shown="真" w397 {
                    tunnel: w401 -> [_ w404]
                    frame False {
                    }
                    frame True {
                      # "4°后重置指示灯状态"
                      n191 = local read "θi"() -> (w408:dbl)
                      n192 = Subtract(x=w404, y=w408) -> (x-y=w409:dbl)
                      n193 = Absolute Value(x=w409) -> (abs(x)=w407:dbl)
                      n194 = Greater?(x=w407, y=15.0) -> (0:w405:bool)
                      n195 = case shown="真" w405 {
                        frame False {
                        }
                        frame True {
                          w410 = FALSE ("Δw1>C")
                          n196 = local write "Δw1>C"(w410) -> ()
                          n197 = local write "Δw2>C"(w410) -> ()
                          n198 = local write "θi"(0.0 ("θ")) -> ()
                        }
                      }
                    }
                  }
                }
              }
            }
            frame #11 {
              n199 = local write "正在测量"(FALSE) -> ()
            }
          }
          n200 = Build Array(w143, w142, w141, w140, w136) -> (w134:dbl[])
          n201 = local read "结果展示"() -> (w133:dbl[][])
          n202 = Insert Into Array(array=w133, new element=w134) -> (→"结果展示":dbl[][])  [unwired: 2 in]
        }
        n203 = Path To String(path=w97) -> (string=w106:string)
        n204 = Concatenate Strings(w106, "循环汇总" ("字符串"), ".xls" ("字符串")) -> (w105:string)
        n205 = VISA Close(VISA resource name=w121, error in (no error)=w120) -> (error out=→"output control error":errorcluster)
        n206 = VISA Close(VISA resource name=w124, error in (no error)=w123) -> (error out=→"照明光error out":errorcluster)
        n207 = String To Path(string=w105) -> (path=w104:path)
        n208 = call-poly <vilib>:"Write Delimited Spreadsheet.vi"("file path (dialog if empty)"=w104, "format (%.3f)"="%.16f", "2D data"=w100, "append to file? (new file:F)"=TRUE ("append to file? (F)"), "transpose? (no:F)"=FALSE ("transpose? (F)")) -> ()  [unwired: 9 in, 2 out]
        n209 = local write "结果展示"(dbl[][] [] ("结果展示")) -> ()
      }
    }
    n210 = event shown="[1] \"低电平持续输出\": 值改变" {
      selector: _ -> [_ _]
      dyn-events: _ -> [_ _]
      timeout: u32 0 ("Time") -> [_ _]
      tunnel: "低电平持续输出" -> [_ w482]
      event Timeout {
        n211 = event-data() -> ()  [unwired: 1 in, 2 out]
      }
      event "低电平持续输出": Value Change {
        w486 = " :SOUR1\n :SOUR2"  # Channel
        n212 = event-data() -> ()  [unwired: 1 in, 6 out]
        n213 = local read "channel输出口"() -> (w487:i32)
        n214 = Pick Line(multi-line string=w486, line index=w487) -> (output string=w485:string)  [unwired: 1 in]
        n215 = local read "VISA 信号发生器"() -> (w490:refnum<visa-resource-name>)
        n216 = VISA Open(VISA resource name=w490) -> (VISA resource name=w489:refnum<visa-resource-name>, error out=w488:errorcluster)  [unwired: 4 in]
        n217 = stacked-sequence {
          seq-local: [w496 _ _ _ _ _ _ _ _ _ _ _ _] -> [_ _ w511 _ _ _ _ _ _ _ _ _ _]
          seq-local: [w495 _ _ _ _ _ _ _ _ _ _ _ _] -> [_ _ w510 _ _ _ _ _ _ _ _ _ _]
          seq-local: [_ _ w509 _ _ _ _ _ _ _ _ _ _] -> [_ _ _ _ w514 _ _ _ _ _ _ _ _]
          seq-local: [_ _ w508 _ _ _ _ _ _ _ _ _ _] -> [_ _ _ _ w515 _ _ _ _ _ _ _ _]
          seq-local: [_ _ _ _ w523 _ _ _ _ _ _ _ _] -> [_ _ _ _ _ _ w534 _ _ _ _ _ _]
          seq-local: [_ _ _ _ w522 _ _ _ _ _ _ _ _] -> [_ _ _ _ _ _ w533 _ _ _ _ _ _]
          seq-local: [_ _ _ _ _ _ w527 _ _ _ _ _ _] -> [_ _ _ _ _ _ _ _ w537 _ _ _ _]
          seq-local: [_ _ _ _ _ _ w526 _ _ _ _ _ _] -> [_ _ _ _ _ _ _ _ w536 _ _ _ _]
          seq-local: [_ _ _ _ _ _ _ _ w540 _ _ _ _] -> [_ _ _ _ _ _ _ _ _ _ w551 _ _]
          seq-local: [_ _ _ _ _ _ _ _ w539 _ _ _ _] -> [_ _ _ _ _ _ _ _ _ _ w550 _ _]
          seq-local: [_ _ _ _ _ _ _ _ _ _ w548 _ _] -> [_ _ _ _ _ _ _ _ _ _ _ _ w565]
          seq-local: [_ _ _ _ _ _ _ _ _ _ w547 _ _] -> [_ _ _ _ _ _ _ _ _ _ _ _ w564]
          tunnel: w489 -> [w501 _ _ _ _ _ _ _ _ _ _ _ _]
          tunnel: w488 -> [w494 _ _ _ _ _ _ _ _ _ _ _ _]
          tunnel: w485 -> [w493 _ w507 _ w520 _ w531 _ w541 _ w554 _ _]
          tunnel: [_ _ _ _ _ _ _ _ _ _ _ _ w563] -> w484
          tunnel: [_ _ _ _ _ _ _ _ _ _ _ _ w561] -> w483
          tunnel: w482 -> [_ _ _ _ _ _ _ _ _ _ _ _ w562]
          frame #0 {
            w498 = " PULSe"  # Function Command
            n218 = local read "输出信号波形"() -> (w492:u16)
            n219 = Concatenate Strings(w493, ":FUNC" ("string (\"\")")) -> (w499:string)
            n220 = Pick Line(string ("")=w499, multi-line string=w498, line index=w492) -> (output string=w497:string)
            n221 = VISA Write(VISA resource name=w501, write buffer=w497, error in (no error)=w494) -> (VISA resource name out=w496:refnum<visa-resource-name>, error out=w495:errorcluster)  [unwired: 1 out]
          }
          frame #1 {
            n222 = Wait (ms)(milliseconds to wait=u32 150) -> ()  [unwired: 1 out]
          }
          frame #2 {
            n223 = Number To Fractional String(use system decimal point (T)=TRUE ("使用系统小数点(T)"), number=1.0 ("数字")) -> (F-format string=w505:string)  [unwired: 2 in]
            n224 = Concatenate Strings ("连接字符串")(w507, ":VOLTage：HIGH ", w505) -> (w504:string)
            n225 = VISA Write(VISA resource name=w511, write buffer=w504, error in (no error)=w510) -> (VISA resource name out=w509:refnum<visa-resource-name>, error out=w508:errorcluster)  [unwired: 1 out]
          }
          frame #3 {
            n226 = Wait (ms)(milliseconds to wait=u32 150) -> ()  [unwired: 1 out]
          }
          frame #4 {
            # "1 电压偏置"
            n227 = Number To Fractional String(use system decimal point (T)=TRUE ("使用系统小数点(T)"), number=0.0 ("数字")) -> (F-format string=w518:string)  [unwired: 2 in]
            n228 = Concatenate Strings(w520, ":VOLTage:LOW ", w518) -> (w519:string)
            n229 = VISA Write(VISA resource name=w514, write buffer=w519, error in (no error)=w515) -> (VISA resource name out=w523:refnum<visa-resource-name>, error out=w522:errorcluster)  [unwired: 1 out]
          }
          frame #5 {
            n230 = Wait (ms)(milliseconds to wait=u32 150) -> ()  [unwired: 1 out]
          }
          frame #6 {
            n231 = local read "channel输出口"() -> (w529:i32)
            n232 = Pick Line(multi-line string=":OUTP1:IMPedance \n:OUTP2:IMPedance " ("write buffer"), line index=w529) -> (output string=w528:string)  [unwired: 1 in]
            n233 = Concatenate Strings ("连接字符串")(w531, w528, "INFINITY") -> (w532:string)
            n234 = VISA Write(VISA resource name=w534, write buffer=w532, error in (no error)=w533) -> (VISA resource name out=w527:refnum<visa-resource-name>, error out=w526:errorcluster)  [unwired: 1 out]
          }
          frame #7 {
            n235 = Wait (ms)(milliseconds to wait=u32 150) -> ()  [unwired: 1 out]
          }
          frame #8 {
            n236 = Number To Fractional String(use system decimal point (T)=TRUE ("使用系统小数点(T)"), number=0.0 ("数字")) -> (F-format string=w544:string)  [unwired: 2 in]
            n237 = Concatenate Strings(w541, ":PULSe:DELay ", w544) -> (w542:string)
            n238 = VISA Write(VISA resource name=w537, write buffer=w542, error in (no error)=w536) -> (VISA resource name out=w540:refnum<visa-resource-name>, error out=w539:errorcluster)  [unwired: 1 out]
          }
          frame #9 {
            n239 = Wait (ms)(milliseconds to wait=u32 150) -> ()  [unwired: 1 out]
          }
          frame #10 {
            w555 = ":LEADing\n:TRAiling "  # Channel
            w559 = ":PULSe:TRANsition"  # VOLTage:Offset
            n240 = local read "上升下降沿"() -> (w556:i32)
            n241 = Pick Line(multi-line string=w555, line index=w556) -> (output string=w552:string)  [unwired: 1 in]
            n242 = Number To Fractional String(use system decimal point (T)=TRUE ("使用系统小数点(T)"), number=0.0 ("数字")) -> (F-format string=w553:string)  [unwired: 2 in]
            n243 = Concatenate Strings(w554, w559, w552, w553) -> (w557:string)
            n244 = VISA Write(VISA resource name=w551, write buffer=w557, error in (no error)=w550) -> (VISA resource name out=w548:refnum<visa-resource-name>, error out=w547:errorcluster)  [unwired: 1 out]
          }
          frame #11 {
            n245 = Wait (ms)(milliseconds to wait=u32 150) -> ()  [unwired: 1 out]
          }
          frame #12 {
            n246 = case shown="假" w562 {
              tunnel: w565 -> [w573 w574]
              tunnel: [w572 w581] -> w561
              tunnel: w564 -> [w571 w579]
              tunnel: [w570 w580] -> w563
              frame True {
                n247 = local write "Output"(TRUE ("布尔")) -> ()
                n248 = local read "channel输出口"() -> (w567:i32)
                n249 = Pick Line(multi-line string=":OUTP1 ON\n:OUTP2 ON" ("write buffer"), line index=w567) -> (output string=w566:string)  [unwired: 1 in]
                n250 = VISA Write(VISA resource name=w573, write buffer=w566, error in (no error)=w571) -> (VISA resource name out=w570:refnum<visa-resource-name>, error out=w572:errorcluster)  [unwired: 1 out]
              }
              frame False {
                n251 = local read "channel输出口"() -> (w576:i32)
                n252 = Pick Line(multi-line string=":OUTP1 OFF\n:OUTP2 OFF" ("write buffer"), line index=w576) -> (output string=w575:string)  [unwired: 1 in]
                n253 = VISA Write(VISA resource name=w574, write buffer=w575, error in (no error)=w579) -> (VISA resource name out=w580:refnum<visa-resource-name>, error out=w581:errorcluster)  [unwired: 1 out]
                n254 = local write "Output"(FALSE ("布尔")) -> ()
              }
            }
          }
        }
        n255 = VISA Close(VISA resource name=w484, error in (no error)=w483) -> (error out=→"output control error  4":errorcluster)
      }
    }
    n256 = event shown="[1] \"Enable\": 值改变" {
      selector: _ -> [_ _]
      dyn-events: _ -> [_ _]
      timeout: u32 0 ("Time") -> [_ _]
      tunnel: "Enable" -> [_ w457]
      event Timeout {
        n257 = event-data() -> ()  [unwired: 1 in, 2 out]
      }
      event "Enable": Value Change {
        n258 = event-data() -> ()  [unwired: 1 in, 6 out]
        n259 = local read "VISA 信号发生器"() -> (w453:refnum<visa-resource-name>)
        n260 = VISA Open(VISA resource name=w453) -> (VISA resource name=w456:refnum<visa-resource-name>, error out=w459:errorcluster)  [unwired: 4 in]
        n261 = stacked-sequence {
          tunnel: w457 -> [w464 _]
          tunnel: w459 -> [w463 _]
          tunnel: w456 -> [w462 _]
          tunnel: [w461 _] -> w455
          tunnel: [w460 _] -> w454
          frame #0 {
            n262 = case shown="真" w464 {
              tunnel: w462 -> [w472 w480]
              tunnel: [w471 w479] -> w460
              tunnel: w463 -> [w470 w477]
              tunnel: [w469 w478] -> w461
              frame True {
                n263 = local write "Output"(TRUE ("布尔")) -> ()
                n264 = local read "channel输出口"() -> (w466:i32)
                n265 = Pick Line(multi-line string=":OUTP1 ON\n:OUTP2 ON" ("write buffer"), line index=w466) -> (output string=w465:string)  [unwired: 1 in]
                n266 = VISA Write(VISA resource name=w472, write buffer=w465, error in (no error)=w470) -> (VISA resource name out=w469:refnum<visa-resource-name>, error out=w471:errorcluster)  [unwired: 1 out]
              }
              frame False {
                n267 = local read "channel输出口"() -> (w474:i32)
                n268 = Pick Line(multi-line string=":OUTP1 OFF\n:OUTP2 OFF" ("write buffer"), line index=w474) -> (output string=w473:string)  [unwired: 1 in]
                n269 = VISA Write(VISA resource name=w480, write buffer=w473, error in (no error)=w477) -> (VISA resource name out=w478:refnum<visa-resource-name>, error out=w479:errorcluster)  [unwired: 1 out]
                n270 = local write "Output"(FALSE ("布尔")) -> ()
              }
            }
          }
          frame #1 {
            n271 = Wait (ms)(milliseconds to wait=u32 150) -> ()  [unwired: 1 out]
          }
        }
        n272 = VISA Close(VISA resource name=w455, error in (no error)=w454) -> (error out=→"output control error  5":errorcluster)
      }
    }
    n273 = event shown="[1] \"Enable 2\": 值改变" {
      selector: _ -> [_ _]
      dyn-events: _ -> [_ _]
      timeout: u32 0 ("Time") -> [_ _]
      tunnel: "Enable 2" -> [_ w27]
      event Timeout {
        n274 = event-data() -> ()  [unwired: 1 in, 2 out]
      }
      event "Enable 2": Value Change {
        n275 = event-data() -> ()  [unwired: 1 in, 6 out]
        n276 = Not(x=w27) -> (.not. x?=w26:bool)
        n277 = local read "VISA 信号发生器"() -> (w28:refnum<visa-resource-name>)
        n278 = VISA Open(VISA resource name=w28) -> (VISA resource name=w31:refnum<visa-resource-name>, error out=w32:errorcluster)  [unwired: 4 in]
        n279 = stacked-sequence {
          tunnel: w26 -> [w37 _]
          tunnel: w32 -> [w36 _]
          tunnel: w31 -> [w35 _]
          tunnel: [w34 _] -> w30
          tunnel: [w33 _] -> w29
          frame #0 {
            n280 = case shown="真" w37 {
              tunnel: w35 -> [w46 w57]
              tunnel: [w45 w56] -> w33
              tunnel: w36 -> [w44 w54]
              tunnel: [w43 w55] -> w34
              frame True {
                n281 = local read "channel输出口"() -> (w39:i32)
                n282 = local write "Output 2"(FALSE ("布尔")) -> ()
                n283 = case shown="1" w39 {
                  tunnel: [1 0] -> w38
                  frame 0, Default {
                  }
                  frame 1 {
                  }
                }
                n284 = Pick Line(multi-line string=":OUTP1 ON\n:OUTP2 ON" ("write buffer"), line index=w38) -> (output string=w40:string)  [unwired: 1 in]
                n285 = VISA Write(VISA resource name=w46, write buffer=w40, error in (no error)=w44) -> (VISA resource name out=w43:refnum<visa-resource-name>, error out=w45:errorcluster)  [unwired: 1 out]
              }
              frame False {
                n286 = local read "channel输出口"() -> (w50:i32)
                n287 = case shown="1" w50 {
                  tunnel: [1 0] -> w49
                  frame 0, Default {
                  }
                  frame 1 {
                  }
                }
                n288 = Pick Line(multi-line string=":OUTP1 OFF\n:OUTP2 OFF" ("write buffer"), line index=w49) -> (output string=w51:string)  [unwired: 1 in]
                n289 = VISA Write(VISA resource name=w57, write buffer=w51, error in (no error)=w54) -> (VISA resource name out=w55:refnum<visa-resource-name>, error out=w56:errorcluster)  [unwired: 1 out]
                n290 = local write "Output 2"(TRUE ("布尔")) -> ()
              }
            }
          }
          frame #1 {
            n291 = Wait (ms)(milliseconds to wait=u32 150) -> ()  [unwired: 1 out]
          }
        }
        n292 = VISA Close(VISA resource name=w30, error in (no error)=w29) -> ()  [unwired: 1 out]
      }
    }
    n293 = case shown="真" "设置参数" {
      frame False {
      }
      frame True {
        w588 = " :SOUR1\n :SOUR2"  # Channel
        n294 = local read "VISA 信号发生器"() -> (w590:refnum<visa-resource-name>)
        n295 = local read "channel输出口"() -> (w589:i32)
        n296 = case shown="1" w589 {
          tunnel: [1 0] -> w582
          frame 0, Default {
          }
          frame 1 {
          }
        }
        n297 = VISA Open(VISA resource name=w590) -> (VISA resource name=w593:refnum<visa-resource-name>, error out=w594:errorcluster)  [unwired: 4 in]
        n298 = Pick Line(multi-line string=w588, line index=w582) -> (output string=w583:string)  [unwired: 1 in]
        n299 = Pick Line(multi-line string=w588, line index=w589) -> (output string=w591:string)  [unwired: 1 in]
        n300 = stacked-sequence {
          seq-local: [w690 _ _ _ _ _ _ _ _ _ _ _ _ _ _] -> [_ _ w705 _ _ _ _ _ _ _ _ _ _ _ _]
          seq-local: [w689 _ _ _ _ _ _ _ _ _ _ _ _ _ _] -> [_ _ w704 _ _ _ _ _ _ _ w743 _ _ _ _]
          seq-local: [_ _ w703 _ _ _ _ _ _ _ _ _ _ _ _] -> [_ _ _ _ w714 _ _ _ _ _ _ _ _ _ _]
          seq-local: [_ _ w702 _ _ _ _ _ _ _ _ _ _ _ _] -> [_ _ _ _ w713 _ _ _ _ _ _ _ _ _ _]
          seq-local: [_ _ _ _ w712 _ _ _ _ _ _ _ _ _ _] -> [_ _ _ _ _ _ w720 _ _ _ _ _ _ _ _]
          seq-local: [_ _ _ _ w709 _ _ _ _ _ _ _ _ _ _] -> [_ _ _ _ _ _ w719 _ _ _ _ _ _ _ _]
          seq-local: [_ _ _ _ _ _ w727 _ _ _ _ _ _ _ _] -> [_ _ _ _ _ _ _ _ w738 _ _ _ _ _ _]
          seq-local: [_ _ _ _ _ _ w726 _ _ _ _ _ _ _ _] -> [_ _ _ _ _ _ _ _ w737 _ _ _ _ _ _]
          seq-local: [_ _ _ _ _ _ _ _ w731 _ _ _ _ _ _] -> [_ _ _ _ _ _ _ _ _ _ w744 _ _ _ _]
          seq-local: [_ _ _ _ _ _ _ _ w730 _ _ _ _ _ _] -> [_ _ _ _ _ _ _ _ _ _ _ _ _ _ _]
          seq-local: [_ _ _ _ _ _ _ _ _ _ w740 _ _ _ _] -> [_ _ _ _ _ _ _ _ _ _ _ _ w754 _ _]
          seq-local: [_ _ _ _ _ _ _ _ _ _ w741 _ _ _ _] -> [_ _ _ _ _ _ _ _ _ _ _ _ w753 _ _]
          seq-local: [_ _ _ _ _ _ _ _ _ _ _ _ w752 _ _] -> [_ _ _ _ _ _ _ _ _ _ _ _ _ _ w765]
          seq-local: [_ _ _ _ _ _ _ _ _ _ _ _ w751 _ _] -> [_ _ _ _ _ _ _ _ _ _ _ _ _ _ w764]
          tunnel: w593 -> [w695 _ _ _ _ _ _ _ _ _ _ _ _ _ _]
          tunnel: w594 -> [w688 _ _ _ _ _ _ _ _ _ _ _ _ _ _]
          tunnel: w591 -> [w687 _ w701 _ w708 _ w724 _ w735 _ w745 _ w755 _ w768]
          tunnel: [_ _ _ _ _ _ _ _ _ _ _ _ _ _ w763] -> w587
          tunnel: [_ _ _ _ _ _ _ _ _ _ _ _ _ _ w762] -> w586
          frame #0 {
            w692 = " PULSe"  # Function Command
            n301 = local read "输出信号波形"() -> (w686:u16)
            n302 = Concatenate Strings(w687, ":FUNC" ("string (\"\")")) -> (w693:string)
            n303 = Pick Line(string ("")=w693, multi-line string=w692, line index=w686) -> (output string=w691:string)
            n304 = VISA Write(VISA resource name=w695, write buffer=w691, error in (no error)=w688) -> (VISA resource name out=w690:refnum<visa-resource-name>, error out=w689:errorcluster)  [unwired: 1 out]
          }
          frame #1 {
            n305 = Wait (ms)(milliseconds to wait=u32 150) -> ()  [unwired: 1 out]
          }
          frame #2 {
            n306 = Number To Fractional String(use system decimal point (T)=TRUE ("使用系统小数点(T)"), number="低电平/V") -> (F-format string=w699:string)  [unwired: 2 in]
            n307 = Concatenate Strings ("连接字符串")(w701, ":VOLTage:LOW ", w699) -> (w698:string)
            n308 = VISA Write(VISA resource name=w705, write buffer=w698, error in (no error)=w704) -> (VISA resource name out=w703:refnum<visa-resource-name>, error out=w702:errorcluster)  [unwired: 1 out]
          }
          frame #3 {
            n309 = Wait (ms)(milliseconds to wait=u32 150) -> ()  [unwired: 1 out]
          }
          frame #4 {
            # "1 频率"
            n310 = Concatenate Strings(w708, ":FREQ ") -> (w715:string)
            n311 = Format Into String ("格式化写入字符串")(initial string=w715, "频率/Hz") -> (resulting string=w716:string)  [unwired: 2 in, 1 out]
            n312 = VISA Write(VISA resource name=w714, write buffer=w716, error in (no error)=w713) -> (VISA resource name out=w712:refnum<visa-resource-name>, error out=w709:errorcluster)  [unwired: 1 out]
          }
          frame #5 {
            n313 = Wait (ms)(milliseconds to wait=u32 150) -> ()  [unwired: 1 out]
          }
          frame #6 {
            n314 = Number To Fractional String(use system decimal point (T)=TRUE ("使用系统小数点(T)"), number="高电平/V") -> (F-format string=w721:string)  [unwired: 2 in]
            n315 = Concatenate Strings(w724, ":VOLTage:HIGH ", w721) -> (w723:string)
            n316 = VISA Write(VISA resource name=w720, write buffer=w723, error in (no error)=w719) -> (VISA resource name out=w727:refnum<visa-resource-name>, error out=w726:errorcluster)  [unwired: 1 out]
          }
          frame #7 {
            n317 = Wait (ms)(milliseconds to wait=u32 150) -> ()  [unwired: 1 out]
          }
          frame #8 {
            n318 = local read "channel输出口"() -> (w733:i32)
            n319 = Pick Line(multi-line string=":OUTP1:IMPedance \n:OUTP2:IMPedance " ("write buffer"), line index=w733) -> (output string=w732:string)  [unwired: 1 in]
            n320 = Concatenate Strings ("连接字符串")(w735, w732, "INFINITY") -> (w736:string)
            n321 = VISA Write(VISA resource name=w738, write buffer=w736, error in (no error)=w737) -> (VISA resource name out=w731:refnum<visa-resource-name>, error out=w730:errorcluster)  [unwired: 1 out]
          }
          frame #9 {
            n322 = Wait (ms)(milliseconds to wait=u32 150) -> ()  [unwired: 1 out]
          }
          frame #10 {
            n323 = Number To Fractional String(use system decimal point (T)=TRUE ("使用系统小数点(T)"), number="占空比/%") -> (F-format string=w747:string)  [unwired: 2 in]
            n324 = Concatenate Strings(w745, ":PULSe:DCYCle ", w747) -> (w742:string)
            n325 = VISA Write(VISA resource name=w744, write buffer=w742, error in (no error)=w743) -> (VISA resource name out=w740:refnum<visa-resource-name>, error out=w741:errorcluster)  [unwired: 1 out]
          }
          frame #11 {
            n326 = Wait (ms)(milliseconds to wait=u32 150) -> ()  [unwired: 1 out]
          }
          frame #12 {
            n327 = Number To Fractional String(use system decimal point (T)=TRUE ("使用系统小数点(T)"), number="延时/s") -> (F-format string=w758:string)  [unwired: 2 in]
            n328 = Concatenate Strings(w755, ":PULSe:DELay ", w758) -> (w756:string)
            n329 = VISA Write(VISA resource name=w754, write buffer=w756, error in (no error)=w753) -> (VISA resource name out=w752:refnum<visa-resource-name>, error out=w751:errorcluster)  [unwired: 1 out]
          }
          frame #13 {
            n330 = Wait (ms)(milliseconds to wait=u32 150) -> ()  [unwired: 1 out]
          }
          frame #14 {
            w769 = ":LEADing\n:TRAiling "  # Channel
            w774 = ":PULSe:TRANsition"  # VOLTage:Offset
            n331 = local read "上升下降沿"() -> (w770:i32)
            n332 = Pick Line(multi-line string=w769, line index=w770) -> (output string=w766:string)  [unwired: 1 in]
            n333 = Number To Fractional String(use system decimal point (T)=TRUE ("使用系统小数点(T)"), number="上升下降沿/s") -> (F-format string=w767:string)  [unwired: 2 in]
            n334 = Concatenate Strings(w768, w774, w766, w767) -> (w771:string)
            n335 = VISA Write(VISA resource name=w765, write buffer=w771, error in (no error)=w764) -> (VISA resource name out=w763:refnum<visa-resource-name>, error out=w762:errorcluster)  [unwired: 1 out]
          }
        }
        n336 = stacked-sequence {
          seq-local: [w601 _ _ _ _ _ _ _ _ _ _ _ _ _ _] -> [_ _ w616 _ _ _ _ _ _ _ _ _ _ _ _]
          seq-local: [w600 _ _ _ _ _ _ _ _ _ _ _ _ _ _] -> [_ _ w615 _ _ _ _ _ _ _ w654 _ _ _ _]
          seq-local: [_ _ w614 _ _ _ _ _ _ _ _ _ _ _ _] -> [_ _ _ _ w625 _ _ _ _ _ _ _ _ _ _]
          seq-local: [_ _ w613 _ _ _ _ _ _ _ _ _ _ _ _] -> [_ _ _ _ w624 _ _ _ _ _ _ _ _ _ _]
          seq-local: [_ _ _ _ w623 _ _ _ _ _ _ _ _ _ _] -> [_ _ _ _ _ _ w631 _ _ _ _ _ _ _ _]
          seq-local: [_ _ _ _ w620 _ _ _ _ _ _ _ _ _ _] -> [_ _ _ _ _ _ w630 _ _ _ _ _ _ _ _]
          seq-local: [_ _ _ _ _ _ w638 _ _ _ _ _ _ _ _] -> [_ _ _ _ _ _ _ _ w649 _ _ _ _ _ _]
          seq-local: [_ _ _ _ _ _ w637 _ _ _ _ _ _ _ _] -> [_ _ _ _ _ _ _ _ w648 _ _ _ _ _ _]
          seq-local: [_ _ _ _ _ _ _ _ w643 _ _ _ _ _ _] -> [_ _ _ _ _ _ _ _ _ _ w655 _ _ _ _]
          seq-local: [_ _ _ _ _ _ _ _ w642 _ _ _ _ _ _] -> [_ _ _ _ _ _ _ _ _ _ _ _ _ _ _]
          seq-local: [_ _ _ _ _ _ _ _ _ _ w651 _ _ _ _] -> [_ _ _ _ _ _ _ _ _ _ _ _ w665 _ _]
          seq-local: [_ _ _ _ _ _ _ _ _ _ w652 _ _ _ _] -> [_ _ _ _ _ _ _ _ _ _ _ _ w664 _ _]
          seq-local: [_ _ _ _ _ _ _ _ _ _ _ _ w663 _ _] -> [_ _ _ _ _ _ _ _ _ _ _ _ _ _ w678]
          seq-local: [_ _ _ _ _ _ _ _ _ _ _ _ w662 _ _] -> [_ _ _ _ _ _ _ _ _ _ _ _ _ _ w677]
          tunnel: w587 -> [w606 _ _ _ _ _ _ _ _ _ _ _ _ _ _]
          tunnel: w586 -> [w599 _ _ _ _ _ _ _ _ _ _ _ _ _ _]
          tunnel: w583 -> [w598 _ w612 _ w619 _ w635 _ w646 _ w656 _ w666 _ w673]
          tunnel: [_ _ _ _ _ _ _ _ _ _ _ _ _ _ w676] -> w585
          tunnel: [_ _ _ _ _ _ _ _ _ _ _ _ _ _ w675] -> w584
          tunnel: w582 -> [_ _ _ _ _ _ _ _ w640 _ _ _ _ _ _]
          frame #0 {
            w603 = " PULSe"  # Function Command
            n337 = Concatenate Strings(w598, ":FUNC" ("string (\"\")")) -> (w604:string)
            n338 = Pick Line(string ("")=w604, multi-line string=w603, line index="输出信号波形 2") -> (output string=w602:string)
            n339 = VISA Write(VISA resource name=w606, write buffer=w602, error in (no error)=w599) -> (VISA resource name out=w601:refnum<visa-resource-name>, error out=w600:errorcluster)  [unwired: 1 out]
          }
          frame #1 {
            n340 = Wait (ms)(milliseconds to wait=u32 150) -> ()  [unwired: 1 out]
          }
          frame #2 {
            n341 = Number To Fractional String(use system decimal point (T)=TRUE ("使用系统小数点(T)"), number="低电平/V 2") -> (F-format string=w610:string)  [unwired: 2 in]
            n342 = Concatenate Strings ("连接字符串")(w612, ":VOLTage:LOW ", w610) -> (w609:string)
            n343 = VISA Write(VISA resource name=w616, write buffer=w609, error in (no error)=w615) -> (VISA resource name out=w614:refnum<visa-resource-name>, error out=w613:errorcluster)  [unwired: 1 out]
          }
          frame #3 {
            n344 = Wait (ms)(milliseconds to wait=u32 150) -> ()  [unwired: 1 out]
          }
          frame #4 {
            # "1 频率"
            n345 = Concatenate Strings(w619, ":FREQ ") -> (w626:string)
            n346 = Format Into String ("格式化写入字符串")(initial string=w626, "频率/Hz 2") -> (resulting string=w627:string)  [unwired: 2 in, 1 out]
            n347 = VISA Write(VISA resource name=w625, write buffer=w627, error in (no error)=w624) -> (VISA resource name out=w623:refnum<visa-resource-name>, error out=w620:errorcluster)  [unwired: 1 out]
          }
          frame #5 {
            n348 = Wait (ms)(milliseconds to wait=u32 150) -> ()  [unwired: 1 out]
          }
          frame #6 {
            n349 = Number To Fractional String(use system decimal point (T)=TRUE ("使用系统小数点(T)"), number="高电平/V 2") -> (F-format string=w632:string)  [unwired: 2 in]
            n350 = Concatenate Strings(w635, ":VOLTage:HIGH ", w632) -> (w634:string)
            n351 = VISA Write(VISA resource name=w631, write buffer=w634, error in (no error)=w630) -> (VISA resource name out=w638:refnum<visa-resource-name>, error out=w637:errorcluster)  [unwired: 1 out]
          }
          frame #7 {
            n352 = Wait (ms)(milliseconds to wait=u32 150) -> ()  [unwired: 1 out]
          }
          frame #8 {
            n353 = Pick Line(multi-line string=":OUTP1:IMPedance \n:OUTP2:IMPedance " ("write buffer"), line index=w640) -> (output string=w644:string)  [unwired: 1 in]
            n354 = Concatenate Strings ("连接字符串")(w646, w644, "INFINITY") -> (w647:string)
            n355 = VISA Write(VISA resource name=w649, write buffer=w647, error in (no error)=w648) -> (VISA resource name out=w643:refnum<visa-resource-name>, error out=w642:errorcluster)  [unwired: 1 out]
          }
          frame #9 {
            n356 = Wait (ms)(milliseconds to wait=u32 150) -> ()  [unwired: 1 out]
          }
          frame #10 {
            n357 = Number To Fractional String(use system decimal point (T)=TRUE ("使用系统小数点(T)"), number="占空比/% 2") -> (F-format string=w658:string)  [unwired: 2 in]
            n358 = Concatenate Strings(w656, ":PULSe:DCYCle ", w658) -> (w653:string)
            n359 = VISA Write(VISA resource name=w655, write buffer=w653, error in (no error)=w654) -> (VISA resource name out=w651:refnum<visa-resource-name>, error out=w652:errorcluster)  [unwired: 1 out]
          }
          frame #11 {
            n360 = Wait (ms)(milliseconds to wait=u32 150) -> ()  [unwired: 1 out]
          }
          frame #12 {
            n361 = Number To Fractional String(use system decimal point (T)=TRUE ("使用系统小数点(T)"), number="延时/s 2") -> (F-format string=w669:string)  [unwired: 2 in]
            n362 = Concatenate Strings(w666, ":PULSe:DELay ", w669) -> (w667:string)
            n363 = VISA Write(VISA resource name=w665, write buffer=w667, error in (no error)=w664) -> (VISA resource name out=w663:refnum<visa-resource-name>, error out=w662:errorcluster)  [unwired: 1 out]
          }
          frame #13 {
            n364 = Wait (ms)(milliseconds to wait=u32 150) -> ()  [unwired: 1 out]
          }
          frame #14 {
            w681 = ":LEADing\n:TRAiling "  # Channel
            w685 = ":PULSe:TRANsition"  # VOLTage:Offset
            n365 = Pick Line(multi-line string=w681, line index="上升下降沿 2") -> (output string=w679:string)  [unwired: 1 in]
            n366 = Number To Fractional String(use system decimal point (T)=TRUE ("使用系统小数点(T)"), number="上升下降沿/s 2") -> (F-format string=w680:string)  [unwired: 2 in]
            n367 = Concatenate Strings(w673, w685, w679, w680) -> (w682:string)
            n368 = VISA Write(VISA resource name=w678, write buffer=w682, error in (no error)=w677) -> (VISA resource name out=w676:refnum<visa-resource-name>, error out=w675:errorcluster)  [unwired: 1 out]
          }
        }
        n369 = VISA Close(VISA resource name=w585, error in (no error)=w584) -> (error out=→"configure error out":errorcluster)
      }
    }
    n370 = event shown="[1] \"照明光\": 值改变" {
      selector: _ -> [_ _]
      dyn-events: _ -> [_ _]
      timeout: 0 -> [_ _]
      tunnel: "照明光" -> [_ w61]
      event Timeout {
        n371 = event-data() -> ()  [unwired: 1 in, 3 out]
      }
      event "照明光": Value Change {
        n372 = event-data() -> ()  [unwired: 1 in, 6 out]
        n373 = local read "stop bits (10: 1 bit)"() -> (w74:u16)
        n374 = local read "parity (0:none)"() -> (w73:enum16{"None", "Odd", "Even", "Mark", "Space"})
        n375 = local read "照明光VISA"() -> (w70:refnum<visa-resource-name>)
        n376 = local read "baud rate"() -> (w71:u32)
        n377 = local read "data bits (8)"() -> (w72:u16)
        n378 = call-poly "VISA Configure Serial Port"("VISA resource name"=w70, "baud rate (9600)"=w71, "data bits (8)"=w72, "parity (0:none)"=w73, "stop bits (10: 1 bit)"=w74) -> ("VISA resource name out"=w67:refnum<visa-resource-name>, "error out"=w66:errorcluster)  [unwired: 9 in]
        n379 = call <vilib>:"Simple Error Handler.vi"("error in (no error)"=w66) -> ()  [unwired: 4 in, 5 out]
        n380 = VISA Open(access mode=0, error in (no error)=w66, VISA resource name=w67) -> (VISA resource name=w69:refnum<visa-resource-name>, error out=w68:errorcluster)  [unwired: 2 in]
        n381 = stacked-sequence {
          tunnel: w69 -> [w79]
          tunnel: w68 -> [w78]
          tunnel: [w77] -> w64
          tunnel: [w76] -> w65
          tunnel: w61 -> [w75]
          frame #0 {
            n382 = case shown="假" w75 {
              tunnel: w79 -> [w85 w95]
              tunnel: [w83 w94] -> w77
              tunnel: w78 -> [w84 w93]
              tunnel: [w82 w92] -> w76
              frame False {
                n383 = Concatenate Strings(" \u0001\u0001¢", "\r") -> (w86:string)
                n384 = VISA Write(VISA resource name=w85, write buffer=w86, error in (no error)=w84) -> (VISA resource name out=w83:refnum<visa-resource-name>, error out=w82:errorcluster)  [unwired: 1 out]
                n385 = Wait (ms)(milliseconds to wait=50) -> ()  [unwired: 1 out]
              }
              frame True {
                w88 = " \u0001\u0000¡"  # Channel
                n386 = Wait (ms)(milliseconds to wait=50) -> ()  [unwired: 1 out]
                n387 = Concatenate Strings(w88, "\r") -> (w89:string)
                n388 = VISA Write(VISA resource name=w95, write buffer=w89, error in (no error)=w93) -> (VISA resource name out=w94:refnum<visa-resource-name>, error out=w92:errorcluster)  [unwired: 1 out]
              }
            }
          }
        }
        n389 = VISA Close(VISA resource name=w64, error in (no error)=w65) -> (error out=w63:errorcluster)
        n390 = call <vilib>:"Simple Error Handler.vi"("error in (no error)"=w63) -> ()  [unwired: 4 in, 5 out]
      }
    }
  }
  n391 = flat-sequence {
    frame #0 {
      "Backlight" <- i32[][] [] ("Backlight")
    }
    frame #1 {
      w776 = FALSE
      # "删除背景光控件\n初始值设定"
      n392 = local write "cut backlight"(w776) -> ()
      "backlight" <- w776
    }
  }
  n393 = stacked-sequence {
    seq-local: [_ _ _ w797 _ _ _ _] -> [_ _ _ _ w815 w835 w838 w1040]
    seq-local: [_ _ _ w796 _ _ _ _] -> [_ _ _ _ w816 w836 w837 w1041]
    frame #0 {
      # "initialize all variables"
      n394 = property on="initialize" class="Bool"("Désactivé"=u8 0) -> ()  [unwired: 2 in, 2 out]
      n395 = property on="Acquire" class="Bool"("Visible"=FALSE) -> ()  [unwired: 2 in, 2 out]
      n396 = property on="Setup" class="Bool"("Visible"=FALSE) -> ()  [unwired: 2 in, 2 out]
      n397 = local write "indicator"("" ("indicator")) -> ()
      n398 = local write "initialized ?"(FALSE ("initialized ?")) -> ()
      n399 = local write "Continuous"(FALSE ("Continuous")) -> ()
      n400 = local write "Close"(FALSE ("Close")) -> ()
      n401 = property on="Device Name" class="Ring (严格)"("Désactivé"=u8 0) -> ()  [unwired: 2 in, 2 out]
      n402 = property on="Continuous" class="Bool (严格)"("Visible"=FALSE) -> ()  [unwired: 2 in, 2 out]
      n403 = local write "Commande tab"(T1."Settings" ("Commande tab")) -> ()
    }
    frame #1 {
      # "Read Uniq ID"
      n404 = stacked-sequence {
        frame #0 {
          n405 = call "read detector uniq-id.vi"() -> ("nbr of components"=w789:i32, "UniqueID"=w788:string[], "Name"=w787:string[])  [unwired: 4 out]
          n406 = for {
            N: w789 -> [_]
            tunnel: w788 -> [w791]
            tunnel: w787 -> [w790]
            n407 = property on="Device Name" class="Ring (严格)"("Chaînes []"=w790) -> ()  [unwired: 2 in, 2 out]
            n408 = property on="Uniques ID" class="Ring (严格)"("Chaînes []"=w791) -> ()  [unwired: 2 in, 2 out]
          }
        }
      }
    }
    frame #2 {
      n409 = while {
        stop <- "initialize" stop-if-true
        n410 = local read "Device Name"() -> (w794:u16)
        n411 = local write "Uniques ID"(w794) -> ()
        n412 = local read "Close"() -> (w792:bool)
        n413 = Stop(stop? (T)=w792) -> ()
        n414 = Wait Until Next ms Multiple(millisecond multiple=u32 100 ("n millisecondes")) -> ()  [unwired: 1 out]
      }
    }
    frame #3 {
      n415 = stacked-sequence {
        tunnel: [_ w804 _ _] -> w797
        tunnel: [_ w803 _ _] -> w796
        frame #0 {
          n416 = local write "indicator"("Initializing ..." ("indicator")) -> ()
        }
        frame #1 {
          n417 = local read "Uniques ID"() -> (w801:u16)
          n418 = property on="Uniques ID" class="Ring (严格)"() -> ("Chaînes []"=w802:string[])  [unwired: 2 in, 2 out]
          n419 = Index Array(array=w802, index=w801) -> (element=w800:string)
          n420 = call "Initialize CCD.vi"("Unique id:"=w800) -> ("activeYPixels"=→"Y Pixels:":i32, "JYCCDLib.IJYCCDReqd"=w803:refnum<k7>, "activeXPixels"=→"X Pixels:":i32, "sortie d'erreur"=w804:errorcluster, "FirmwareVersion"=→"Firmware\nVersion":string)  [unwired: 3 out]
        }
        frame #2 {
          n421 = property on="initialize" class="Bool"("Désactivé"=u8 2) -> ()  [unwired: 2 in, 2 out]
          n422 = property on="Device Name" class="Ring (严格)"("Désactivé"=u8 2) -> ()  [unwired: 2 in, 2 out]
          n423 = local write "Continuous"(FALSE ("Continuous")) -> ()
          n424 = property on="Setup" class="Bool"("Visible"=TRUE) -> ()  [unwired: 2 in, 2 out]
        }
        frame #3 {
          n425 = local write "initialized ?"(TRUE ("initialized ?")) -> ()
          n426 = local write "indicator"("Initialized !" ("indicator")) -> ()
        }
      }
    }
    frame #4 {
      # "Actually not working"
      # "Read ADC and GAIN"
      n427 = case shown="真" "Constante de condition\n(Voir l'aide contextuelle)" {
        tunnel: w816 -> [_ w826]
        tunnel: w815 -> [_ w825]
        frame False {
        }
        frame True {
          # "Read Input supported trigger"
          n428 = call "Trigger - Get Supported Input.vi"("JYCCDLib.IJYCCDReqd"=w826, "Error Input"=w825) -> ("trigAddress"=w820:i32, "eventPtr"=w821:i32, "trigEventString"=w824:string, "trigSigType"=w823:i32, "trigSigTypeString"=w822:string)  [unwired: 4 out]
          n429 = local write "trigSigTypeString"(w822) -> ()
          n430 = local write "trigAddress"(w820) -> ()
          n431 = local write "Trigger Type :"(w821) -> ()
          n432 = local write "trigEventString"(w824) -> ()
          n433 = local write "Signal type :"(w823) -> ()
        }
      }
      n434 = call "Init ADC & Gain.vi"("JYCCDLib.IJYCCDReqd"=w816, "input error"=w815) -> ("ADC Number"=w814:i32[], "ADC description"=w819:string[], "Gain Number"=w817:i32[], "Gain description"=w818:string[])
      n435 = local write "Gain Number"(w817) -> ()
      n436 = local write "ADC Number"(w814) -> ()
      n437 = stacked-sequence {
        tunnel: w819 -> [w827 _]
        tunnel: w818 -> [_ w828]
        frame #0 {
          n438 = property on="ADC" class="Ring (严格)"("Chaînes []"=w827) -> ()  [unwired: 2 in, 2 out]
        }
        frame #1 {
          n439 = property on="GAIN" class="Ring (严格)"("Chaînes []"=w828) -> ()  [unwired: 2 in, 2 out]
        }
      }
    }
    frame #5 {
      # "IS multi Accumulation Supported ?"
      n440 = call "MultiAccu - Is Supported.vi"("Error In"=w835, "JYCCDLib.IJYCCDReqd"=w836) -> ("IsOperatingModeSupported"=w829:bool)  [unwired: 3 out]
      n441 = Select(t=0, s=w829, f=2) -> (s? t:f=w832:i32)
      n442 = Select(t=FALSE, s=w829, f=w829) -> (s? t:f=w831:bool)
      n443 = local write "Multi Accumulation mode:"(w831) -> ()
      n444 = property on="Multi Accumulation mode:" class="Bool (严格)"("Désactivé"=w832) -> ()  [unwired: 2 in, 2 out]
      n445 = property on="Multi Accumulation mode:" class="Bool (严格)"("Désactivé"=w832) -> ()  [unwired: 2 in, 2 out]
    }
    frame #6 {
      n446 = while {
        tunnel: w837 -> [w845]
        tunnel: w838 -> [w844]
        stop <- "Close" stop-if-true
        n447 = local read "Continuous"() -> (w846:bool)
        n448 = case shown="假" "Reformat" {
          frame False {
          }
          frame True {
            n449 = local read "Y Pixels:"() -> (w1018:i32)
            n450 = local read "X Pixels:"() -> (w1020:i32)
            n451 = call "Spectral Reformat CCD area.vi"("Y Pixels:"=w1018, "X Pixels:"=w1020, "numAreas"="Number of Areas :") -> ("areas :"=→"areas :":i32[][])  [unwired: 3 out]
          }
        }
        n452 = local read "Accumulations:"() -> (w841:u16)
        n453 = Or(x="Acquire", y=w846) -> (x .or. y?=w843:bool)
        n454 = case shown="真" w843 {
          tunnel: w845 -> [_ w858]
          tunnel: w844 -> [_ w857]
          tunnel: "Enable InputTriggers :" -> [_ w856]
          tunnel: "Multi Accumulation mode:" -> [_ w855]
          tunnel: w841 -> [_ w854]
          tunnel: "MultiAcqShutterMode" -> [_ w853]
          frame False {
          }
          frame True {
            n455 = stacked-sequence {
              seq-local: [_ _ w871 _ _] -> [_ _ _ w944 _]
              seq-local: [_ _ _ w917 _] -> [_ _ _ _ w984]
              tunnel: w858 -> [_ w860 w875 w943 _]
              tunnel: w857 -> [_ w861 w874 w942 _]
              tunnel: w856 -> [_ w862 _ _ _]
              tunnel: w855 -> [_ _ w873 _ _]
              tunnel: w854 -> [_ _ w872 _ _]
              tunnel: w853 -> [_ _ w870 _ _]
              frame #0 {
                n456 = local write "CCD Busy"(TRUE ("CCD Busy")) -> ()
              }
              frame #1 {
                n457 = case shown="真" w862 {
                  tunnel: w861 -> [w863 w869]
                  tunnel: w860 -> [w864 w868]
                  frame False {
                    n458 = call "Trigger - Disable.vi"("Error In"=w863, "JYCCDLib.IJYCCDReqd"=w864) -> ()  [unwired: 6 out]
                  }
                  frame True {
                    n459 = local read "Trigger Type :"() -> (w865:u16)
                    n460 = local read "Signal type :"() -> (w866:enum16{"TTL Rising Edge", "TTL Falling Edge"})
                    n461 = local read "trigAddress"() -> (w867:i32)
                    n462 = call "Trigger - Enable.vi"("Error In"=w869, "sigType"=w866, "event"=w865, "trigAddress"=w867, "JYCCDLib.IJYCCDReqd"=w868) -> ()  [unwired: 3 out]
                  }
                }
              }
              frame #2 {
                n463 = case shown="真" w873 {
                  selector: w873 -> [_ w904]
                  tunnel: w875 -> [w901 w907]
                  tunnel: w874 -> [w900 w906]
                  tunnel: w872 -> [_ w905]
                  tunnel: [u16 1 ("Accumulations:") w905] -> w871
                  tunnel: w870 -> [_ w903]
                  frame False {
                    n464 = call "MultiAccu - Disable.vi"("Error In"=w900, "JYCCDLib.IJYCCDReqd"=w901) -> ()  [unwired: 4 out]
                  }
                  frame True {
                    n465 = call "MultiAccu - Configure.vi"("JYCCDLib.IJYCCDReqd"=w907, "Cleans Before"="Number of Cleans", "Accumulations:"=w905, "MultiAcqHardwareMode"=w904, "MultiAcqShutterMode"=w903, "Error In"=w906) -> ()  [unwired: 1 in, 9 out]
                  }
                }
                n466 = flat-sequence {
                  frame #0 {
                    n467 = Current VI's Path() -> (path=w881:path)
                    n468 = Get Date/Time In Seconds() -> (seconds since 1Jan1904=w883:timestamp)
                    n469 = Strip Path(path=w881) -> (stripped path=w882:path)  [unwired: 1 out]
                    n470 = Path To String(path=w882) -> (string=w884:string)
                    n471 = Format Date/Time String(time format string (%c)="%m.%d" ("时间格式字符串(%c)"), seconds (now)=w883) -> (date/time string=w890:string)  [unwired: 1 in]
                    n472 = Concatenate Strings(w884, "\\Save\\" ("字符串"), w890) -> (w885:string)
                    n473 = String To Path(string=w885) -> (path=w886:path)
                    n474 = call <vilib>:"Check if File or Folder Exists.vi"("path"=w886) -> ("file or folder exists?"=w887:bool, "dup path"=w889:path)  [unwired: 8 in, 1 out]
                    n475 = case shown="真" w887 {
                      tunnel: [w897 w898] -> w888
                      tunnel: w889 -> [w896 w898]
                      tunnel: w890 -> [w895 _]
                      frame False {
                        n476 = Create Folder(prompt (Create Folder)=w895, path (use dialog)=w896) -> (created path=w897:path)  [unwired: 1 in, 2 out]
                      }
                      frame True {
                      }
                    }
                    n477 = Format Date/Time String(time format string (%c)="%y%m%d%H%M%S " ("时间格式字符串(%c)"), seconds (now)=w883) -> (date/time string=w893:string)  [unwired: 1 in]
                    n478 = Path To String(path=w888) -> (string=w891:string)
                    n479 = Concatenate Strings(w891, "\\" ("字符串")) -> (w892:string)
                    n480 = Concatenate Strings(w892, w893) -> (w880:string)
                    n481 = String To Path(string=w880) -> (path=→"最终存储路径 2":path)
                  }
                }
              }
              frame #3 {
                n482 = local read "cut backlight"() -> (w931:bool)
                n483 = local read "backlight"() -> (w930:bool)
                n484 = call "MultiAccu - Acquire spectral.vi"("error in"=w942, "Accumulations:"=w944, "ShutterOpen"="ShutterOpen", "JYCCDLib.IJYCCDReqd"=w943) -> ("Acq Time(ms)"=→"Acq Time(ms)":u32, "Array Out"=w941:i32[][][])  [unwired: 1 out]
                n485 = And(x=w931, y=w930) -> (x .and. y?=w932:bool)
                n486 = call "Array reset dimension.vi"("Area Number"="Area Number to Display", "Array In"=w941) -> ("Array Out"=w933:i32[][])
                n487 = case shown="真" w932 {
                  tunnel: [w980 w981] -> w934
                  tunnel: w933 -> [w980 w982]
                  frame False {
                  }
                  frame True {
                    n488 = local read "Backlight"() -> (w983:i32[][])
                    n489 = Subtract(x=w982, y=w983) -> (x-y=w981:i32[][])
                  }
                }
                n490 = local read "波长范围"() -> (w909:dbl[])
                n491 = local write "Data"(w933) -> ()
                n492 = Index Array(array=w934, index (row)=0 ("禁用的索引 (列)")) -> (element=w935:i32[])  [unwired: 1 in]
                n493 = Reverse 1D Array(array=w935) -> (reversed array=w918:i32[])
                n494 = call "转换至动态数据2"("Array"=w909) -> ("Dynamic Data Type"=w937:dynamicdata)  [unwired: 3 in]
                n495 = call "转换至动态数据"("Array"=w918) -> ("Dynamic Data Type"=w938:dynamicdata)  [unwired: 3 in]
                n496 = call <vilib>:"Median Filter.vi"("left rank"=6, "X"=w918) -> ("Filtered X"=w923:dbl[])  [unwired: 8 in, 1 out]
                n497 = call "Build XY Graph2"("Y Input"=w938, "X Input"=w937) -> ("XY Graph"=w936:cluster{"Y":dbl[], "Y":dbl[]}[])  [unwired: 8 in, 1 out]
                n498 = Subtract(x="拟合终点", y="拟合起点") -> (x-y=w912:i32)
                n499 = local write "Spectrum"(w936) -> ()
                n500 = local read "滤波阈值"() -> (w927:dbl)
                n501 = Array Subset(array=w909, index="拟合起点", length=w912) -> (w915:dbl[])
                n502 = local read "拟合参数"() -> (w908:dbl[])
                n503 = In Range and Coerce(upper limit=w927, x=w923, lower limit=-100.0) -> (In Range?=w926:bool[])  [unwired: 1 out]
                n504 = Not(x=w926) -> (.not. x?=w920:bool[])
                n505 = local read "滤波阈值"() -> (w922:dbl)
                n506 = local write "范围内？"(w926) -> ()
                n507 = local read "X Pixels:"() -> (w924:i32)
                n508 = Or Array Elements(Boolean array=w920) -> (logical OR=w925:bool)
                n509 = case shown="真" w925 {
                  tunnel: w924 -> [_ w967]
                  tunnel: w923 -> [w963 w966]
                  tunnel: [w963 w965] -> w911
                  tunnel: w922 -> [_ w964]
                  frame False {
                  }
                  frame True {
                    n510 = for {
                      N: w967 -> [_]
                      tunnel: w966 -> [w971] mode=indexing
                      tunnel: [w970] -> w965 mode=indexing
                      shift-right: [w970] -> _
                      shift-left: _ -> [w969]
                      tunnel: w964 -> [w968]
                      n511 = Greater?(x=w971, y=w968) -> (0:w973:bool)
                      n512 = Less?(x=w971, y=-100.0) -> (x < y?=w974:bool)
                      n513 = Or(x=w973, y=w974) -> (x .or. y?=w972:bool)
                      n514 = case shown="真" w972 {
                        tunnel: w971 -> [w976 _]
                        tunnel: [w976 w978] -> w970
                        tunnel: w969 -> [_ w979]
                        frame False {
                        }
                        frame True {
                          n515 = call <vilib>:"Median Filter PtByPt.vi"("rank"=5, "x"=w979) -> ("Filtered x"=w978:dbl)  [unwired: 2 in, 1 out]
                        }
                      }
                    }
                  }
                }
                n516 = Array Subset(array=w911, index="拟合起点", length=w912) -> (w914:dbl[])
                n517 = Bundle("波长范围"=w909, "Filtered X"=w911) -> (w910:cluster{"波长范围 ":dbl[], "Filtered X":dbl[]})  [unwired: 1 in]
                n518 = case shown="真" "是否拟合" {
                  tunnel: w914 -> [w947 w953]
                  tunnel: w915 -> [_ w952]
                  tunnel: [w947 w951] -> w929
                  tunnel: w910 -> [_ w949]
                  frame False {
                  }
                  frame True {
                    n519 = call "转换至动态数据7"("Array"=w953) -> ("Dynamic Data Type"=w958:dynamicdata)  [unwired: 3 in]
                    n520 = call "转换至动态数据8"("Array"=w952) -> ("Dynamic Data Type"=w959:dynamicdata)  [unwired: 3 in]
                    n521 = call "曲线拟合2"("Locations"=w959, "Signals"=w958) -> ("best fit"=w956:dynamicdata, "non-linear coefficients"=w957:dynamicdata)  [unwired: 5 in, 3 out]
                    n522 = call "从动态数据转换3"("Dynamic Data Type"=w957) -> ("Array"=w960:dbl[])  [unwired: 3 in]
                    n523 = call "从动态数据转换4"("Dynamic Data Type"=w956) -> ("Array"=w951:dbl[])  [unwired: 3 in]
                    n524 = Index Array(array=w960, index #1=0 ("索引"), index #2=1 ("索引")) -> (element #1=w962:dbl, element #2=w961:dbl)
                    n525 = local write "拟合参数"(w960) -> ()
                    n526 = local write "xc"(w962) -> ()
                    n527 = Bundle(w952, "Array"=w951) -> (w950:cluster{dbl[], "Array":dbl[]})  [unwired: 1 in]
                    n528 = local write "w"(w961) -> ()
                    n529 = Build Array(w949, w950) -> (→"best fit":cluster{"波长范围 ":dbl[], "Array":dbl[]}[])
                  }
                }
                n530 = Build Array(w915, w918, w929, w908) -> (w917:dbl[][])
              }
              frame #4 {
                n531 = case shown="真" "是否保存" {
                  tunnel: w984 -> [_ w988]
                  frame False {
                  }
                  frame True {
                    n532 = Get Date/Time In Seconds() -> (seconds since 1Jan1904=w1002:timestamp)
                    n533 = Get Date/Time String(date format (0)=enum16{"short", "long", "abbreviated"}."abbreviated" ("日期格式(0)"), seconds (now)=w1002, want seconds? (F)=TRUE ("需要秒？(F)")) -> (date string=w1000:string, time string=w1001:string)
                    n534 = Search and Replace String(replace all?=TRUE ("替换全部？(F)"), input string=w1001, search string=":" ("搜索字符串"), replace string="-" ("替换字符串(\"\")")) -> (result string=w999:string)  [unwired: 4 in, 3 out]
                    n535 = local read "最终存储路径 2"() -> (w1003:path)
                    n536 = Path To String(path=w1003) -> (string=w1006:string)
                    n537 = Concatenate Strings(w1006, w1000, w999, "光谱" ("字符串"), ".xls" ("字符串")) -> (w1005:string)
                    n538 = String To Path(string=w1005) -> (path=w1004:path)
                    n539 = call-poly <vilib>:"Write Delimited Spreadsheet.vi"("file path (dialog if empty)"=w1004, "format (%.3f)"="%.16f", "2D data"=w988, "append to file? (new file:F)"=TRUE ("append to file? (F)"), "transpose? (no:F)"=TRUE ("transpose? (F)")) -> ()  [unwired: 9 in, 2 out]
                  }
                }
                n540 = case shown="真" "Save Backlight" {
                  frame False {
                  }
                  frame True {
                    w1007 = TRUE ("删除背景光")
                    n541 = local read "Data"() -> (w1009:i32[][])
                    n542 = local write "Backlight"(w1009) -> ()
                    n543 = local write "cut backlight"(w1007) -> ()
                    n544 = local write "backlight"(w1007) -> ()
                    n545 = local write "Save Backlight"(FALSE ("Save Backlight")) -> ()
                  }
                }
                n546 = local write "CCD Busy"(FALSE ("CCD Busy")) -> ()
              }
            }
          }
        }
        n547 = case shown="假" "Setup" {
          tunnel: w844 -> [_ w1023]
          tunnel: w845 -> [_ w1022]
          frame False {
          }
          frame True {
            n548 = stacked-sequence {
              tunnel: w1023 -> [_ w1037 _]
              tunnel: w1022 -> [_ w1025 _]
              frame #0 {
                n549 = local write "indicator"("Setting up the detector" ("indicator")) -> ()
              }
              frame #1 {
                w1035 = 1 items=["JYMCD_ACQ_FORMAT_IMAGE", "JYMCD_ACQ_FORMAT_SCAN"] ("Acquisition type")
                n550 = local read "Gain Number"() -> (w1030:i32[])
                n551 = local read "GAIN"() -> (w1026:u16)
                n552 = local read "ADC Number"() -> (w1031:i32[])
                n553 = local read "ADC"() -> (w1027:u16)
                n554 = Index Array(array=w1030, index=w1026) -> (element=w1028:i32)
                n555 = Index Array(array=w1031, index=w1027) -> (element=w1029:i32)
                n556 = local read "Number of Areas :"() -> (w1033:u16)
                n557 = local read "areas :"() -> (w1034:i32[][])
                n558 = call "Setup CCD.vi"("numAreas"=w1033, "areas :"=w1034, "JYCCDLib.IJYCCDReqd"=w1025, "entrée d'erreur (pas d'erreur)"=w1037, "Acquisition type"=w1035, "Gain"=w1028, "Select ADC"=w1029, "Integration time(ms)"="Integration time (ms) :") -> ("DataSize"=→"DataSize":i32)  [unwired: 1 out]
                "JYCCDLib.IJYCCDReqd" <- w1025
              }
              frame #2 {
                w1038 = TRUE ("Visible")
                n559 = property on="Continuous" class="Bool (严格)"("Visible"=w1038) -> ()  [unwired: 2 in, 2 out]
                n560 = property on="Acquire" class="Bool"("Visible"=w1038) -> ()  [unwired: 2 in, 2 out]
                n561 = local write "indicator"("Ready !" ("indicator")) -> ()
              }
            }
          }
        }
        n562 = case shown="假" "Temperature" {
          tunnel: w845 -> [_ w1012]
          tunnel: w844 -> [_ w1011]
          frame False {
            n563 = property on="temp graph" class="WFChart (严格)"("Visible"=FALSE) -> ()  [unwired: 2 in, 2 out]
          }
          frame True {
            n564 = stacked-sequence {
              tunnel: w1012 -> [_ w1017]
              tunnel: w1011 -> [_ w1016]
              frame #0 {
                n565 = property on="temp graph" class="WFChart (严格)"("Visible"=TRUE) -> ()  [unwired: 2 in, 2 out]
              }
              frame #1 {
                w1015 = u16 0 items=["° Celsius", "Kelvin", "° Farenheit"] ("units")
                n566 = call "read temperature.vi"("entrée d'erreur (pas d'erreur)"=w1016, "units"=w1015, "JYCCDLib.IJYCCDReqd"=w1017) -> ("Current Temperature"=w1014:dbl)
                n567 = local write "temp graph"(w1014) -> ()
              }
            }
          }
        }
        n568 = Wait Until Next ms Multiple(millisecond multiple=u32 50 ("n millisecondes")) -> ()  [unwired: 1 out]
      }
    }
    frame #7 {
      n569 = Close Reference(reference=w1041, error in (no error)=w1040) -> ()  [unwired: 1 out]
    }
  }
  n570 = stacked-sequence {
    seq-local: [_ _ w1051 _ _] -> [_ _ _ w1061 w1066]
    seq-local: [_ _ w1050 _ _] -> [_ _ _ w1060 _]
    seq-local: [_ _ _ w1059 _] -> [_ _ _ _ _]
    frame #0 {
      n571 = call "Get Monos From Config Browser.vi"() -> ("UniqueIDs"=w1046:string[], "Mono ID"=w1047:string[])  [unwired: 3 in, 1 out]
      n572 = Build Cluster Array(w1047, w1046) -> (w1044:cluster{"String":string, "String":string}[])
      n573 = property on="Mono ID" class="CmbBox"("Strings And Values []"=w1044) -> ()  [unwired: 2 in, 2 out]
      n574 = Index Array(array=w1044, index=0) -> (element=w1045:cluster{"String":string, "String":string})
      n575 = Unbundle(w1045) -> ("String"=w1042:string)  [unwired: 1 out]
      "Current UniqueID" <- w1042
      n576 = local write "Mono ID"(w1042) -> ()
    }
    frame #1 {
      n577 = while {
        stop <- "Connect" stop-if-true
        n578 = local read "Mono ID"() -> (w1048:string)
        n579 = local write "Current UniqueID"(w1048) -> ()
      }
    }
    frame #2 {
      n580 = local read "Mono ID"() -> (w1053:string)
      n581 = call "JYInitMono.vi"("Unique ID"=w1053, "Force Init"="Force\nInitialization") -> ("Refnum out"=w1051:refnum<k7>, "Initialized"=→"Initialized JY":bool, "error out"=w1050:errorcluster)  [unwired: 9 in, 2 out]
    }
    frame #3 {
      n582 = call "Show Current Grating.vi"("Refnum in"=w1061, "error in (no error)"=w1060) -> ("Gratings"=w1062:dbl[], "Grating Index"=w1056:i32, "Current Grating"=w1058:dbl, "Current Description"=w1055:string, "error out"=w1059:errorcluster)  [unwired: 5 in, 4 out]
      "Gratings" <- w1062
      n583 = local write "Current Grating"(w1058) -> ()
      n584 = local write "Current Description"(w1055) -> ()
      n585 = Number To Decimal String(number=w1062) -> (decimal integer string=w1064:string[])  [unwired: 1 in]
      n586 = Number To Decimal String(number=w1056) -> (decimal integer string=w1057:string)  [unwired: 1 in]
      n587 = property on="Target Grating" class="CmbBox"("Value"=w1057) -> ()  [unwired: 2 in, 2 out]
      n588 = Build Cluster Array(w1064, string[] ["1", "2", "3"]) -> (w1065:cluster{"Numeric":string, string}[])
      n589 = property on="Target Grating" class="CmbBox"("Strings And Values []"=w1065) -> ()  [unwired: 2 in, 2 out]
    }
    frame #4 {
      n590 = while {
        tunnel: w1066 -> [w1068]
        stop <- w1067 stop-if-true
        n591 = stacked-sequence {
          seq-local: [w1072 _ _ _ _] -> [_ w1079 w1090 _ w1098]
          seq-local: [w1071 _ _ _ _] -> [_ w1078 w1089 _ _]
          seq-local: [_ w1077 _ _ _] -> [_ _ _ _ _]
          seq-local: [_ w1076 _ _ _] -> [_ _ _ _ _]
          seq-local: [_ _ w1082 _ _] -> [_ _ _ _ _]
          seq-local: [_ _ w1081 _ _] -> [_ _ _ w1092 _]
          tunnel: w1068 -> [w1070 _ _ w1093 _]
          frame #0 {
            n592 = call "Show Current Grating.vi"("Refnum in"=w1070) -> ("Grating Index"=→"Grating Index":i32, "Current Grating"=→"Current Grating":dbl, "Current Description"=→"Current Description":string, "error out"=w1071:errorcluster, "JYMONOLib.IJYMonoReqd"=w1072:refnum<k7>)  [unwired: 6 in, 4 out]
          }
          frame #1 {
            n593 = call "JYGetCurrentWL.vi"("error in (no error)"=w1078, "JYMONOLib.IJYMonoReqd"=w1079) -> ("error out"=w1076:errorcluster, "Units"=→"Units":string, "Current WL"=→"Current WL":dbl, "JYMONOLib.IJYMonoReqd 2"=w1077:refnum<k7>)  [unwired: 6 in]
          }
          frame #2 {
            w1087 = u16 1 items=["Entrance", "Exit"] ("Mirror Number")
            w1088 = u16 0 items=["Entrance", "Exit"] ("Mirror Number")
            n594 = call "JYGetMirrorPos.vi"("error in (no error)"=w1089, "Mirror"=w1088, "Refnum In"=w1090) -> ("error out"=w1085:errorcluster, "Current Mirror Position"=→"Entrance Mirror\nPosition":i32, "Refnum Out"=w1086:refnum<k7>)  [unwired: 1 in]
            n595 = call "JYGetMirrorPos.vi"("error in (no error)"=w1085, "Mirror"=w1087, "Refnum In"=w1086) -> ("error out"=w1081:errorcluster, "Current Mirror Position"=→"Exit Mirror\nPosition":i32, "Refnum Out"=w1082:refnum<k7>)  [unwired: 1 in]
          }
          frame #3 {
            w1095 = u16 0 items=["Front Entrance", "Side Entrance", "Front Exit", "Side Exit", "First Intermediate", "Second Intermediate"] ("Slit")
            n596 = call "JYGetSlits.vi"("MonoRefNum IN"=w1093, "Slit"=w1095, "error in (no error)"=w1092) -> ("Units"=→"Units 2":string, "Slit Width"=→"Front Entrance":dbl, "error out"=→"error out":errorcluster)  [unwired: 13 in, 1 out]
          }
          frame #4 {
            n597 = case shown="假" "Move To\nTarget Positions" {
              tunnel: w1098 -> [_ w1099]
              frame False {
              }
              frame True {
                n598 = stacked-sequence {
                  seq-local: [w1101 _ _ _] -> [_ w1107 _ _]
                  seq-local: [_ w1105 _ _] -> [_ _ w1122 _]
                  seq-local: [_ _ w1109 _] -> [_ _ _ w1128]
                  seq-local: [_ _ _ w1125] -> [_ _ _ _]
                  tunnel: w1099 -> [w1103 w1106 w1120 w1129]
                  frame #0 {
                    n599 = property on="Target Grating" class="CmbBox"() -> ("Value"=w1100:string)  [unwired: 2 in, 2 out]
                    n600 = local read "error out"() -> (w1102:errorcluster)
                    n601 = Decimal String To Number(string=w1100) -> (number=w1104:i32)  [unwired: 2 in, 1 out]
                    n602 = call "JYTurret.vi"("error in (no error)"=w1102, "Grating Index"=w1104, "JYMONOLib.IJYMonoReqd"=w1103) -> ("error out"=w1101:errorcluster)  [unwired: 2 out]
                  }
                  frame #1 {
                    # "Move Grating to Target Position"
                    n603 = call "JYMoveToWavelength.vi"("error in (no error)"=w1107, "Target WL"="Target WL", "RefNum In"=w1106) -> ("error out"=w1105:errorcluster)  [unwired: 1 in, 2 out]
                  }
                  frame #2 {
                    w1115 = u16 1 items=["Entrance", "Exit"] ("Mirror Number")
                    w1114 = u16 0 items=["Entrance", "Exit"] ("Mirror Number")
                    w1121 = u16 1 items=["Entrance", "Exit", "Front", "Side"] ("Mirror Number")
                    w1124 = u16 0 items=["Entrance", "Exit", "Front", "Side"] ("Mirror Number")
                    # "Move Mirrors"
                    n604 = call "JYMirrorMove.vi"("error in (no error)"=w1122, "Mirror Position"="Entrance Mirror", "Mirror Number"=w1124, "RefNum In"=w1120) -> ("error out"=w1119:errorcluster)  [unwired: 6 in, 1 out]
                    n605 = call "JYMirrorMove.vi"("error in (no error)"=w1119, "Mirror Position"="Exit Mirror", "Mirror Number"=w1121, "RefNum In"=w1120) -> ("error out"=w1112:errorcluster, "MonoRefNum Out"=w1113:refnum<k7>)  [unwired: 6 in]
                    n606 = call "JYGetMirrorPos.vi"("error in (no error)"=w1112, "Mirror"=w1114, "Refnum In"=w1113) -> ("error out"=w1117:errorcluster, "Current Mirror Position"=w1111:i32, "Refnum Out"=w1116:refnum<k7>)  [unwired: 1 in]
                    n607 = local write "Entrance Mirror\nPosition"(w1111) -> ()
                    n608 = call "JYGetMirrorPos.vi"("error in (no error)"=w1117, "Mirror"=w1115, "Refnum In"=w1116) -> ("error out"=w1109:errorcluster, "Current Mirror Position"=w1110:i32)  [unwired: 1 in, 1 out]
                    n609 = local write "Exit Mirror\nPosition"(w1110) -> ()
                  }
                  frame #3 {
                    w1127 = u16 0 items=["Front Entrance", "Side Entrance", "Front Exit", "Side Exit", "First Intermediate", "Second Intermediate"] ("Slit")
                    # "Set New Slit Positions"
                    n610 = call "JYSlits.vi"("JYMONOLib.IJYMonoReqd"=w1129, "Slit"=w1127, "error in (no error)"=w1128, "Slit Width"="Target\nFront Entrance") -> ("error out"=w1125:errorcluster)  [unwired: 1 in, 1 out]
                  }
                }
              }
            }
          }
        }
        n611 = local read "Close"() -> (w1067:bool)
      }
    }
  }
  n612 = flat-sequence {
    frame #0 {
      n613 = call <vilib>:"Create Report.vi"("window state (normal)"=T3."no change", "report type"=Report_Type."Excel", "template (empty)"=path "D:/desktop/train/TEST1/Save/516中心波长.xlsx") -> ("report out"=w1136:refnum<class "NI_report.lvclass">, "error out"=w1135:errorcluster)  [unwired: 11 in]
      n614 = call-poly <vilib>:"Excel Get Data.vi"("report in"=w1136, "data type"=string[][] [], "error in (no error)"=w1135) -> ("report out"=w1131:refnum<class "NI_report.lvclass">, "data"=w1139:string[][], "error out"=w1130:errorcluster)  [unwired: 10 in]
      n615 = call-dynamic "Dispose Report.vi"("report in"=w1131, "error in (no error)"=w1130) -> ()  [unwired: 13 in, 1 out]
      n616 = Index Array(array=w1139, index (col)=0 ("禁用的索引 (列)")) -> (element=w1141:string[])  [unwired: 1 in]
      n617 = Fract/Exp String To Number(string=w1141) -> (number=→"波长范围":dbl[])  [unwired: 3 in, 1 out]
    }
  }
